vi "User Calibration.vi"(0 "CalStatusTab":T4(tab), 1 "SetDac In Process":bool, 5 "Processed Variables":T3 {"Chamber Temperature" format="%.2f"; "Ambient Temperature" format="%.2f"; "Bath Temperature" format="%.2f"; "Det. Temperature" format="%.2f"; "Detector Chl 4" format="%.2g"; "Detector Chl 3" format="%.2g"; "Ref CO2" format="%.2g"; "Detector Chl 2" format="%.2g"; "Film Temperature" format="%.2f"; "Humidity" format="%.2f"; "Detector Chl 1" format="%.2g"}, 9 "DACSet":u16[](array[numeric]) format="%03x", 11 "time_now":timestamp format="%<%H:%M:%S>T", 12 "Coefficients_In":T2[](array[typedef]) {"Elapsed Time" format="%<%H:%M:%S>t"; "zero_utc" format="%x"; "cal_utc" format="%x"; "Pump Flow Rate" format="%0d"; "Number of Zeroes" format="%0d"; "V2C" format="%0d"; "C2V" format="%0d"; "duration" format="%<%H:%M:%S>t"; "DAC" format="%03x"; "mI" format="%.3g"; "V_(RA,15mA)" format="%0.4f"; "V_(RA,5mA)" format="%0.4f"; "Chamber Temp" format="%.1f"; "Humidity" format="%.1f"}) -> (2 "Cal Fail":bool, 3 "Calibration Complete":bool, 4 "CalStatus Out":u16, 6 "DAC Currents":sgl[](array[numeric]) caption="Currents" format="%.4g", 8 "CalGasTank":u8=5 max=7, 10 "Pump Settings":T1, 14 "Coefficients_Out":T2[](array[typedef]) {"Elapsed Time" format="%<%H:%M:%S>t"; "zero_utc" format="%x"; "cal_utc" format="%x"; "Pump Flow Rate" format="%0d"; "Number of Zeroes" format="%0d"; "V2C" format="%0d"; "C2V" format="%0d"; "duration" format="%<%H:%M:%S>t"; "DAC" format="%03x"; "mI" format="%.3g"; "V_(RA,15mA)" format="%0.4f"; "V_(RA,5mA)" format="%0.4f"; "Chamber Temp" format="%.1f"; "Humidity" format="%.1f"}, 15 "SetDac":bool)   [LabVIEW 2015]
uses:
  <vilib>/Analysis/NI_AALBase.lvlib
  <vilib>/Analysis/baseanly.llb/Mean (DBL).vi
  Controls/Calibration Coefficients.ctl
  Controls/Processed Variables.ctl
  Controls/Pump Settings.ctl
panel:
  out "Error":bool
  out "Index":u16
  out "null array":i16[][](array[numeric])
  out "stage 4 - offset adjust":i16[][](array[numeric])=[[0, 3, 500, 1, 1], [1, 3, 500, 1, 1], [2, 3, 500, 1, 1], [3, 3, 500, 1, 1], [4, 3, 500, 1, 1], [5, 3, 500, 1, 1], [6, 3, 500, 1, 1], [7, 3, 500, 0, 0], [8, 3, 500, 0, 0], [9, 3, 500, 0, 0], [10, 3, 500, 0, 0], [11, 3, 500, 0, 0], [12, 3, 500, 0, 0], [13, 3, 500, 0, 0], [14, 3, 500, 0, 0], [15, 3, 500, 0, 0], [16, 3, 500, 0, 0], [17, 3, 500, 0, 0], [18, 3, 500, 0, 0], [19, 3, 500, 0, 0], [20, 3, 500, 0, 0], [21, 3, 500, 0, 0], [22, 3, 500, 0, 0], [23, 3, 500, 0, 0], [24, 3, 500, 0, 0], [25, 3, 500, 0, 0], [26, 3, 500, 0, 0], [27, 3, 500, 0, 0], [28, 3, 500, 0, 0], [29, 3, 500, 0, 0], [30, 3, 500, 0, 0], [31, 3, 500, 0, 0], [32, 3, 500, 0, 0], [33, 3, 500, 0, 0], [34, 3, 500, 0, 0], [35, 3, 500, 0, 0], [36, 3, 500, 0, 0], [37, 3, 500, 0, 0], [38, 3, 500, 0, 0], [39, 3, 500, 0, 0], [40, 3, 500, 0, 0], [41, 3, 500, 0, 0], [42, 3, 500, 0, 0], [43, 3, 500, 0, 0], [44, 3, 500, 0, 0], [45, 3, 500, 0, 0], [46, 3, 500, 0, 0], [47, 3, 500, 0, 0], [48, 3, 500, 0, 0], [49, 3, 500, 0, 0], [50, 3, 500, 0, 0], [51, 3, 500, 0, 0], [52, 3, 500, 0, 0], [53, 3, 500, 0, 0], [54, 3, 500, 0, 0], [55, 3, 500, 0, 0], [56, 3, 500, 0, 0], [57, 3, 500, 0, 0], [58, 3, 500, 0, 0], [59, 3, 500, 0, 0], [60, 3, 500, 0, 0], [61, 3, 500, 0, 0], [62, 3, 500, 0, 0], [63, 3, 500, 0, 0], [64, 3, 500, 0, 0], [65, 3, 500, 0, 0], [66, 3, 500, 0, 0], [67, 3, 500, 0, 0], [68, 3, 500, 0, 0], [69, 3, 500, 0, 0], [70, 3, 500, 0, 0], [71, 3, 500, 0, 0], [72, 3, 500, 0, 0], [73, 3, 500, 0, 0], [74, 3, 500, 0, 0], [75, 3, 500, 0, 0], [76, 3, 500, 0, 0], [77, 3, 500, 0, 0], [78, 3, 500, 0, 0], [79, 3, 500, 0, 0], [80, 3, 500, 0, 0], [81, 3, 500, 0, 0], [82, 3, 500, 0, 0], [83, 3, 500, 0, 0], [84, 3, 500, 0, 0], [85, 3, 500, 0, 0], [86, 3, 500, 0, 0], [87, 3, 500, 0, 0], [88, 3, 500, 0, 0], [89, 3, 500, 0, 0], [90, 3, 500, 0, 0], [91, 3, 500, 0, 0], [92, 3, 50, 1, 1]]
  out "stage 3 - span":i16[][](array[numeric])=[[0, 3, 500, 0, 1], [1, 3, 500, 0, 1], [2, 3, 500, 0, 1], [3, 3, 500, 0, 1], [4, 3, 500, 0, 1], [5, 3, 500, 0, 1], [6, 3, 50, 0, 1]]
  out "stage 2 - zeroing":i16[][](array[numeric])=[[0, 2, 500, 1, 0], [1, 2, 500, 1, 0], [2, 2, 500, 1, 0], [3, 2, 500, 1, 0], [4, 2, 500, 1, 0], [5, 2, 500, 1, 0], [6, 2, 50, 1, 0]]
  out "stage1 - humidity check":i16[][](array[numeric])=[[0, 1, 500, 1, 0], [1, 1, 50, 1, 0], [2, 1, 50, 1, 0], [3, 1, 50, 1, 0], [4, 1, 50, 1, 0], [5, 1, 50, 1, 0], [6, 1, 100, 0, 1], [7, 1, 150, 0, 1], [8, 1, 200, 0, 1], [9, 1, 250, 1, 0], [10, 1, 300, 1, 1], [0, 1, 350, 0, 0]]
  out "Tcal_Film":dbl format="%.2f"
  out "I_delta":dbl[](array[numeric]) format="%0.4f"
  out "Actual":u16
  in  "Lo Flow":u16=50
  out "Tcal_Det":dbl[](array[numeric]) format="%.2f"
  out "Raw_Humidity":dbl format="%.2f"
  out "Raw Chamber":dbl format="%.2f"
  in  "Quit":bool
  in  "CalFile":path
  in  "Calfiles":string[](array[string])
  out "Reference":dbl format="%.3g"
  out "Tcal_Humidity":dbl format="%.2f"
  in  "Hi Flow Setting":u16=100
  out "Progress Out":u8(slide) scale=0.0..255.0
  in  "Progress":u16(slide) scale=0.0..666.0
  out "Cal Gas":dbl=nan format="%.3g"
  in  "Skip Cal":bool
  in  "OK  7":bool
  in  "Calgas":dbl caption="Calibration Gas Concentration" format="%.2g"
  out "start time":timestamp format="%<%H:%M:%S>T"
  in  "Gas Tank":u8=5
  out "Calibration Message":enum16{"Calibration Is Required - "}(ring)
  in  "Calibration Code":T5(ring)
  out "Stable":bool
  in  "Low Humidity Threshold (%)":u16=60
  in  "Hi Humidity Threshold (%)":u16=90
  in  "Humidity Status":T6(ring)
  out "Stablizing":dbl[][](graph)
  out "Status":bool[](array[boolean])
  out "V2C":u8[](array[numeric])
  out "D'":dbl[](array[numeric]) format="%0.4f"
  out "C'":dbl[](array[numeric]) format="%0.4f"
  out "B'":dbl[](array[numeric]) format="%0.4f"
  out "A'":dbl[](array[numeric]) format="%0.4f"
  out "D":dbl[](array[numeric]) format="%0.4f"
  out "C":dbl[](array[numeric]) format="%0.4f"
  out "B":dbl[](array[numeric]) format="%0.4f"
  out "A":dbl[](array[numeric]) format="%0.4f"
  out "C2V":u8[](array[numeric])
  out "CHANNEL":string[](array[string])
  out "C0FC2V":dbl[](array[numeric]) format="%0.4f"
  out "C6FC2V":dbl[](array[numeric]) format="%0.4f"
  out "TYPE":string
  out "DATE":string
  out "CalFile Selected":path
  out "V_0d(target)":dbl[](array[numeric]) format="%0.4f"
  out "V_6d(target)":dbl[](array[numeric]) format="%0.4f"
  out "V_span(target)":dbl[](array[numeric]) format="%0.4f"
  out "BlueLED 2":bool[](array[boolean]) caption="BlueLED"
  out "DAC scale":dbl[](array[numeric]) format="%.3g"
  out "Zero":dbl[][](graph)
  out "Zero Status":T7(ring)
  out "V_RA(5mA)":dbl[](array[numeric]) format="%0.4f"
  out "V_RA(15mA)":dbl[](array[numeric]) format="%0.4f"
  out "mI":dbl[](array[numeric]) format="%.3g"
  out "delta 2":dbl=nan caption="delta" format="%.3g"
  out "CHANNEL 2":string[](array[string]) caption="CHANNEL"
  out "BlueLED":bool[](array[boolean])
  in  "OK 9":bool
  out "Span Point Calibration":dbl[][](graph)
  out "I_span":dbl[](array[numeric]) format="%0.4f"
  out "Step":i16[](array[numeric])
  out "DAC":u16[](array[numeric]) format="%03x"
  out "V_Span Delta":dbl[](array[numeric]) format="%0.4f"
  out "Span Good":bool[](array[boolean])
  out "I'mBlue":bool[](array[boolean]) caption="BlueLED"
  out "delta":dbl=nan format="%.3g"
  out "Zero Offset":dbl[][](graph)
  in  "OK 10":bool
  out "Calibration Complete -":timestamp format="%<%H:%M:%S\n%m/%d/%y>T"
  out "duration":i16 caption="mins" format="%<%H:%M:%S>t"
  out "V_0d(ImA)":dbl[](array[numeric]) format="%0.4f"
  out "V_6d(ImA)":dbl[](array[numeric]) format="%0.4f"
  out "V_0(adjust)":dbl[](array[numeric]) format="%0.4f"
  out "V_span(adjust)":dbl[](array[numeric]) format="%0.4f"
  out "Gain(adjust)":dbl[](array[numeric]) format="%0.4f"
  out "V_span(ImA)":dbl[](array[numeric]) format="%0.4f"
  out "Tcal_PCB":dbl=nan format="%.2f"
  out "Tcal_Chamber":dbl format="%.2f"
  out "elapsed time":i16 format="%<%H:%M:%S>t"
  out "Count":u8
  # "Channel 1"
  # "Channel 2"
  # "Channel 3"
  # "Channel 4"
  # "Initializing"
  # "1. Please Place Freespira On Base-Station\n \n2. Attach Cannula and Breathe Normally \n \n3. Enter Calibration Gas Concentration \n \n4. Press OK To Begin Calibration Process"
  # "Please Enter Calibration Code"
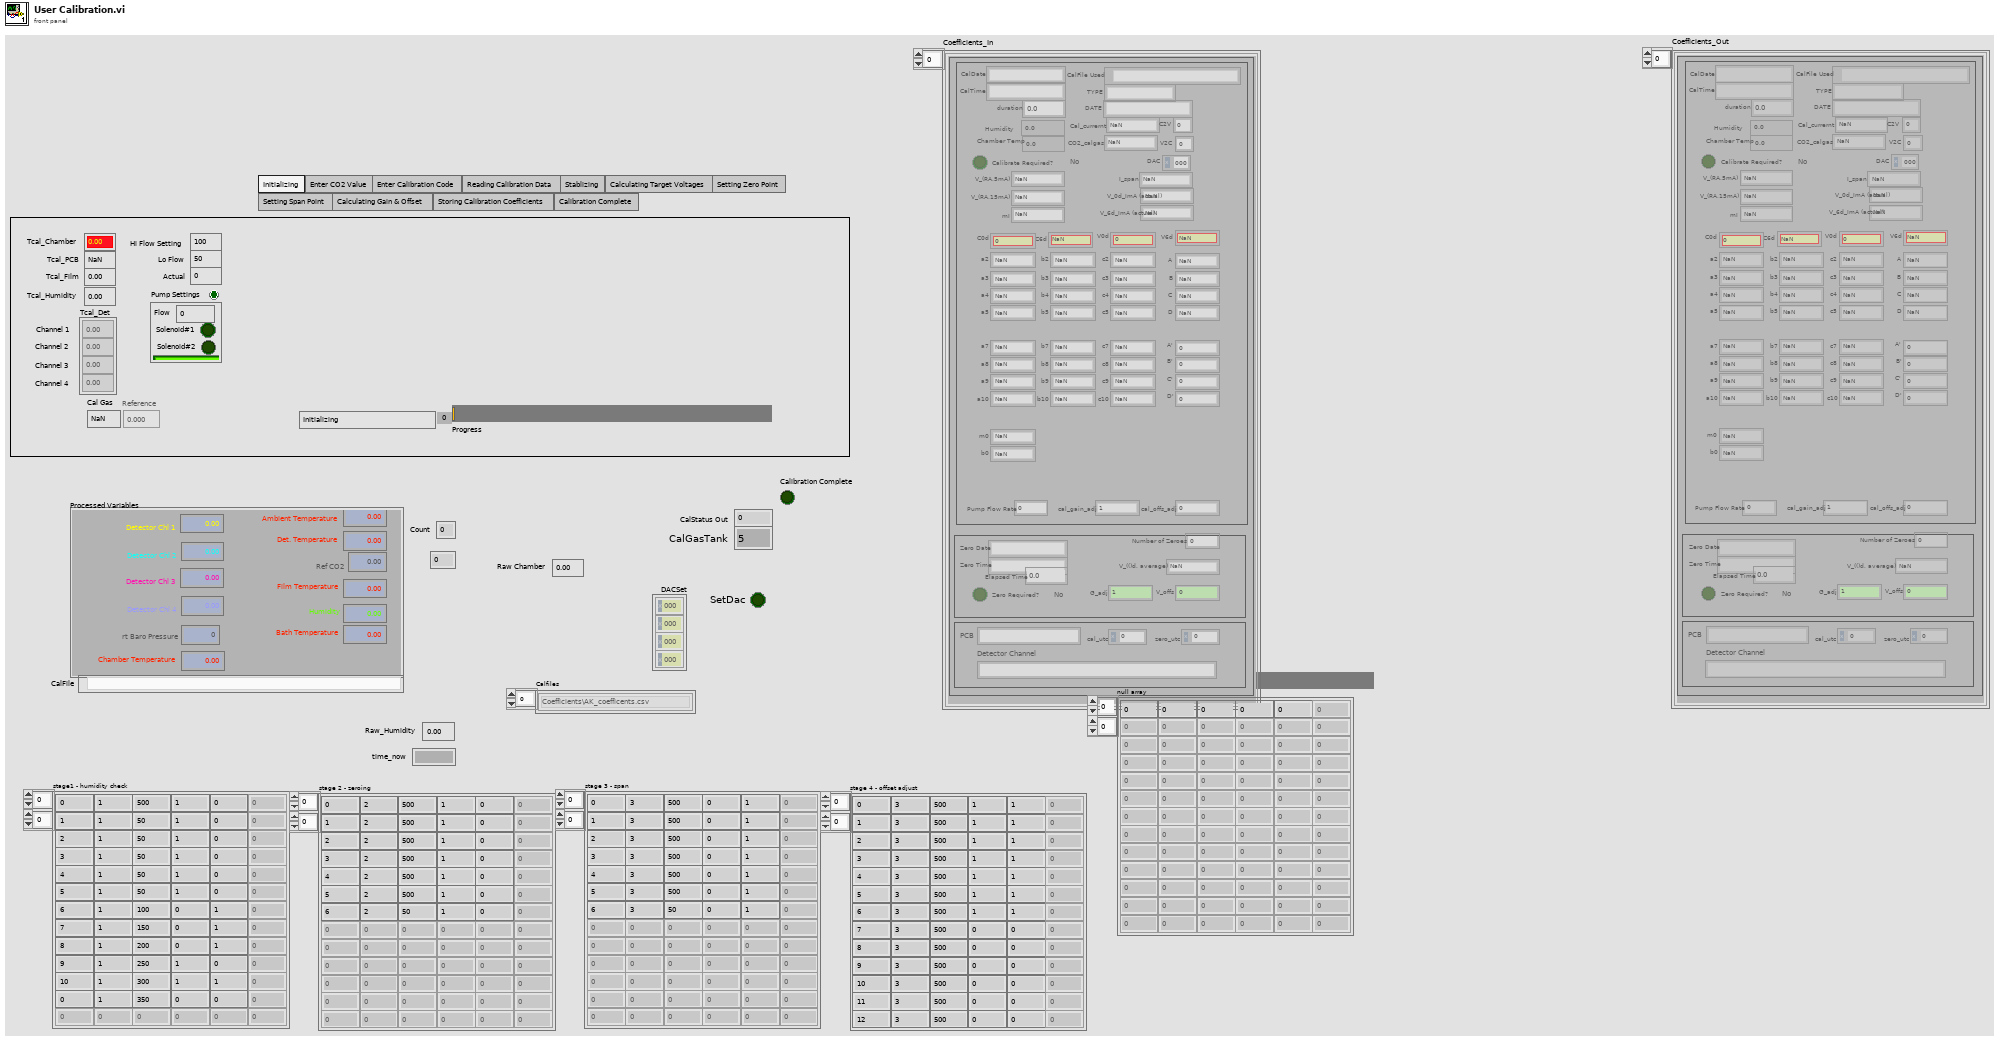
[diagram p1: front panel]
types:
  T1 = typedef "Pump Settings.ctl" = cluster{"Flow":u16, "Solenoid#1":bool, "Solenoid#2":bool, "ignore":bool}
  T2 = typedef "Calibration Coefficients.ctl" = cluster{"CalFile Used":path, "TYPE":string, "DATE":string, "Humidity":sgl, "Chamber Temp":dbl, "CO2_calgas":dbl, "V_(RA,5mA)":dbl, "V_(RA,15mA)":dbl, "mI":dbl, "V_0d_ImA (actual)":dbl, "V_6d_ImA (actual)":dbl, "I_span":dbl, "DAC":u16, "A":dbl, "B":dbl, "C":dbl, "D":dbl, "V6d":dbl, "A'":dbl, "B'":dbl, "C'":dbl, "D'":dbl, "V0d":dbl, "CalDate":string, "CalTime":string, "duration":dbl, "Detector Channel":string, "a2":dbl, "a3":dbl, "a4":dbl, "a5":dbl, "b2":dbl, "c2":dbl, "b3":dbl, "c3":dbl, "b4":dbl, "c4":dbl, "b5":dbl, "c5":dbl, "a7":dbl, "a8":dbl, "a9":dbl, "a10":dbl, "b7":dbl, "b8":dbl, "b9":dbl, "b10":dbl, "c7":dbl, "c8":dbl, "c9":dbl, "c10":dbl, "cal_offs_adj":dbl, "cal_gain_adj":dbl, "C6d":dbl, "C0d":dbl, "Cal_currernt":dbl, "C2V":u16, "V2C":u16, "Zero Date":string, "Zero Time":string, "Number of Zeroes":u16, "V_(()d, average)":dbl, "V_offs ":dbl, "G_adj":dbl, "Pump Flow Rate":u16, "Zero Required? ":bool, "Calibrate Required?":bool, "cal_utc":dbl, "zero_utc":dbl, "Elapsed Time":dbl, "PCB":string, "m0":dbl, "b0":dbl}
  T3 = typedef "Processed Variables.ctl" = cluster{"Detector Chl 1":sgl, "Humidity":dbl, "Film Temperature":dbl, "Detector Chl 2":sgl, "Ref CO2":sgl, "Detector Chl 3":sgl, "Detector Chl 4":sgl, "Det. Temperature":dbl, "Bath Temperature":dbl, "Ambient Temperature":dbl, "rt Baro Pressure":u16, "Chamber Temperature":dbl}
  T4 = enum32{"Initializing", "Enter CO2 Value", "Enter Calibration Code", "Reading Calibration Data", "Stablizing", "Calculating Target Voltages", "Setting Zero Point", "Setting Span Point", "Calculating Gain & Offset", "Storing Calibration Coefficients", "Calibration Complete"}
  T5 = enum8{"", "<User Defined>", "11111 - default", "22222 - MM_1_NS", "33333 - MM_2_S"}
  T6 = enum16{"Waiting For Film to Stabilize", "Film Stable", "Exiting", "Initializing"}
  T7 = enum16{"Setting Zero at 5 mA", "Setting Zero at 15 mA", "Calculating slopes"}
  T8 = enum32{"Invalid", "Standard", "Closed", "Hidden", "Minimized", "Maximized"}
  T9 = enum16{"Waiting For Film to Stabilize", "Film Stable - Press OK to Continue", "Exiting"}
  T10 = enum16{"Waiting For Film to Stabilize", "Film Stable - Press OK to Continue", "Exiting", "Initializing"}
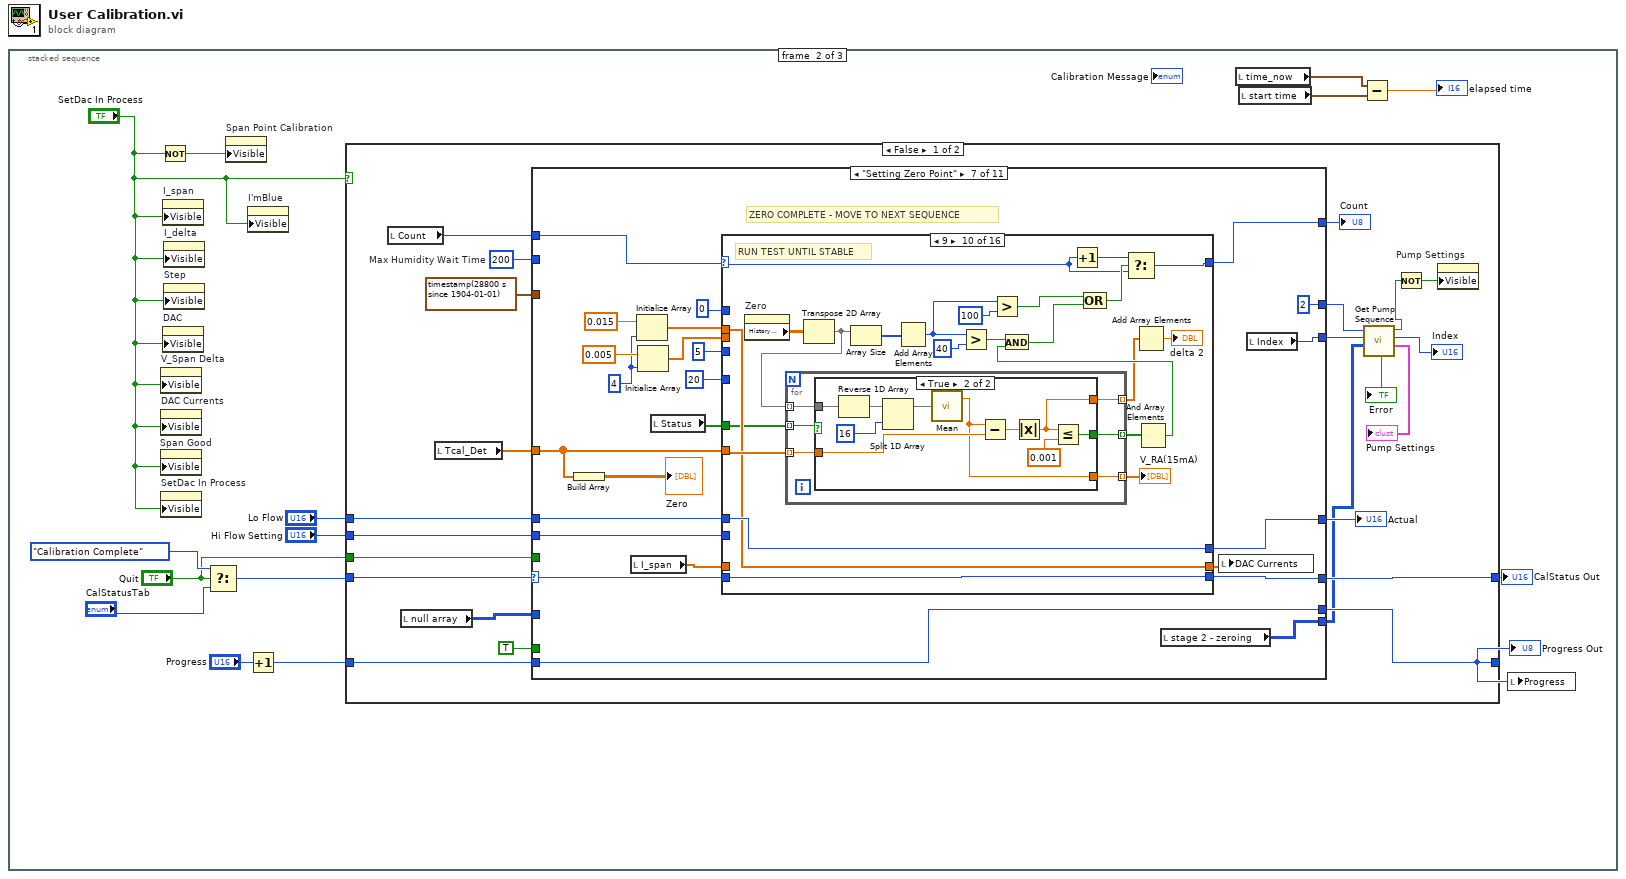
[diagram p0: block diagram]
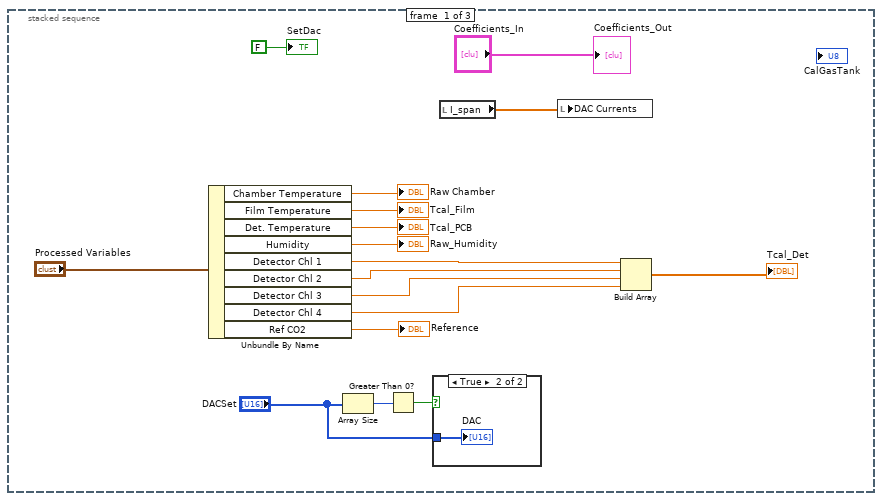
[diagram p2: hidden frame]
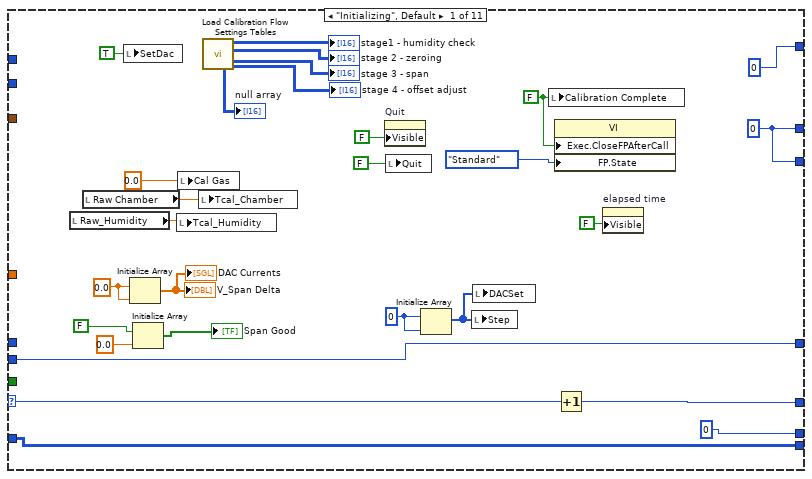
[diagram p4: hidden frame]
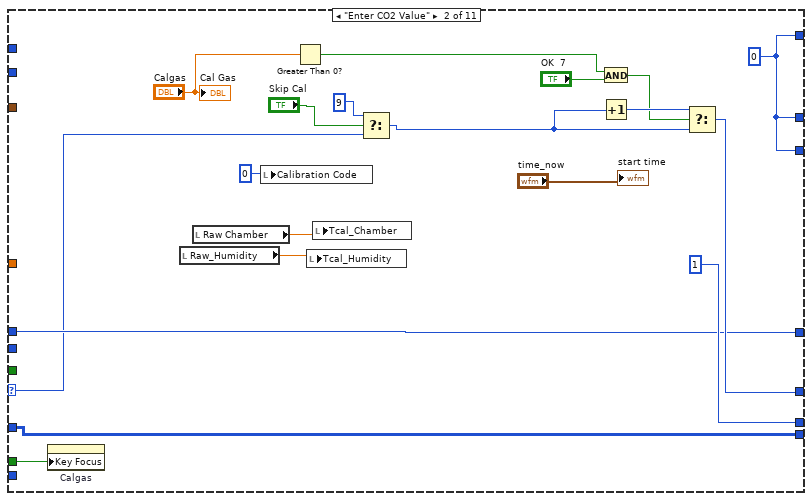
[diagram p5: hidden frame]
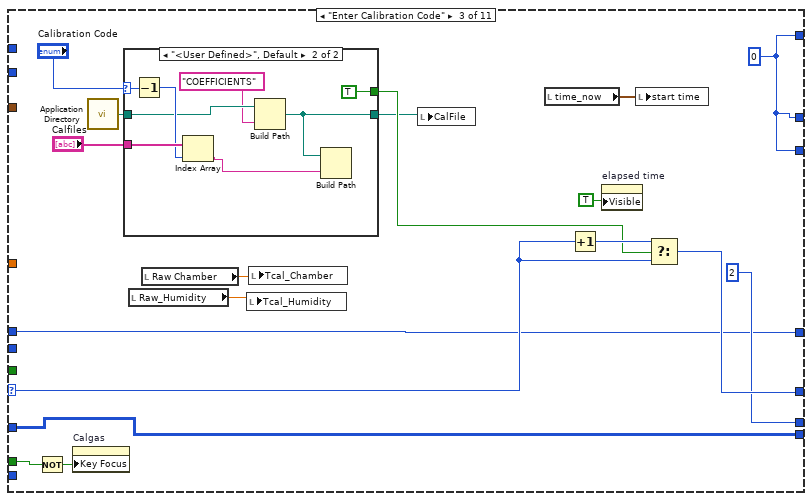
[diagram p6: hidden frame]
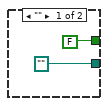
[diagram p7: hidden frame]
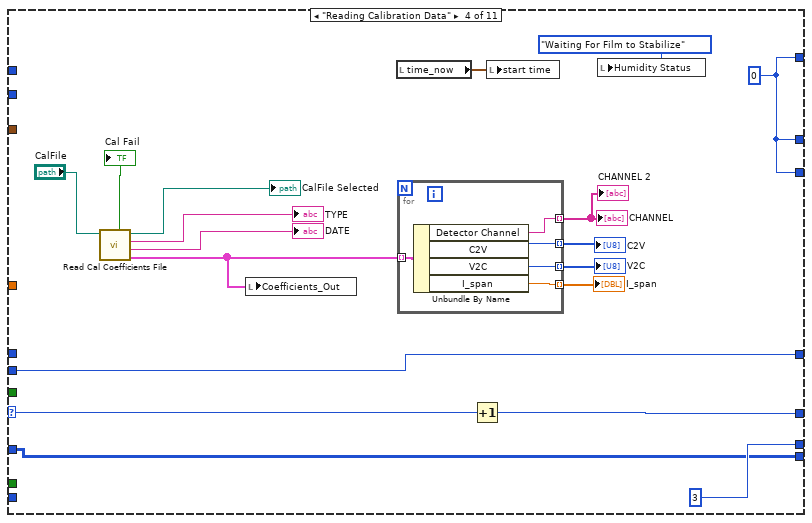
[diagram p8: hidden frame]
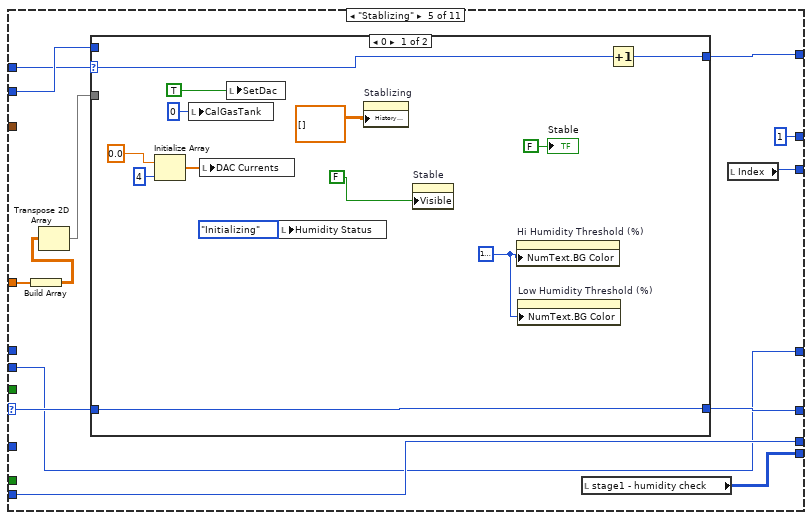
[diagram p9: hidden frame]
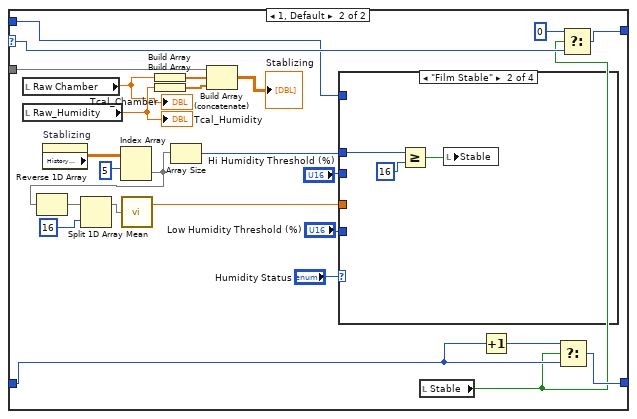
[diagram p10: hidden frame]
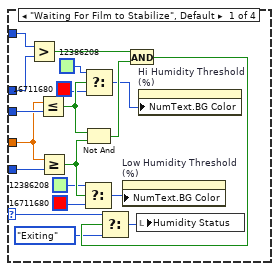
[diagram p11: hidden frame]
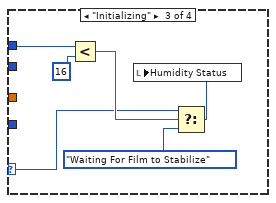
[diagram p12: hidden frame]
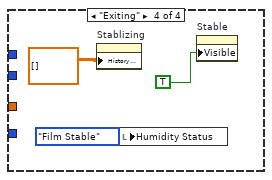
[diagram p13: hidden frame]
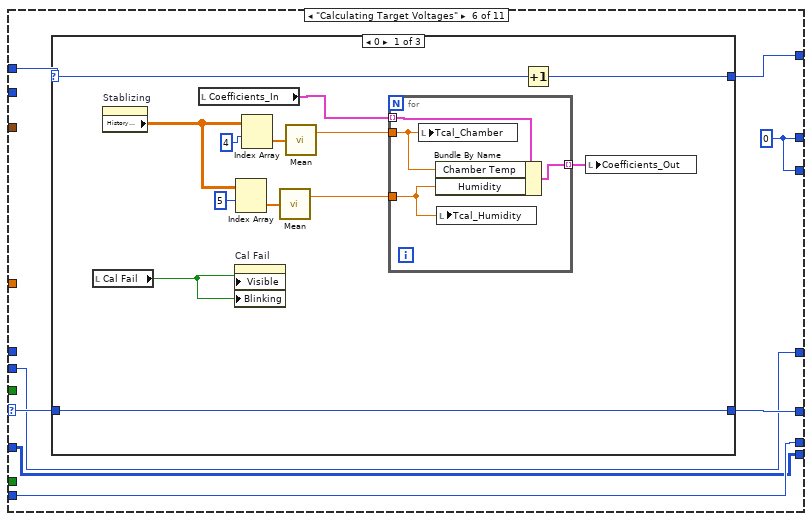
[diagram p14: hidden frame]
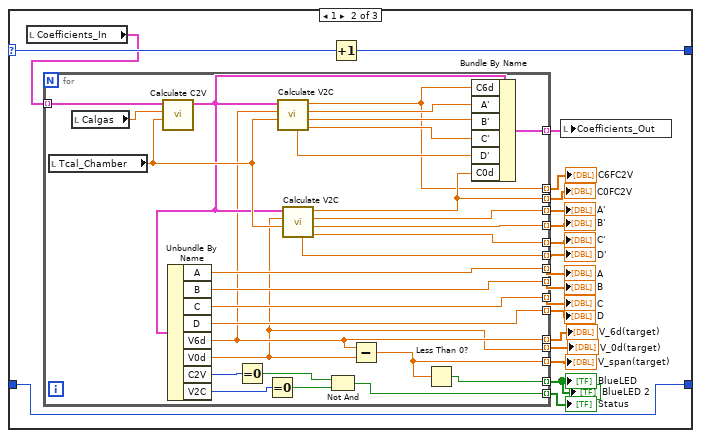
[diagram p15: hidden frame]
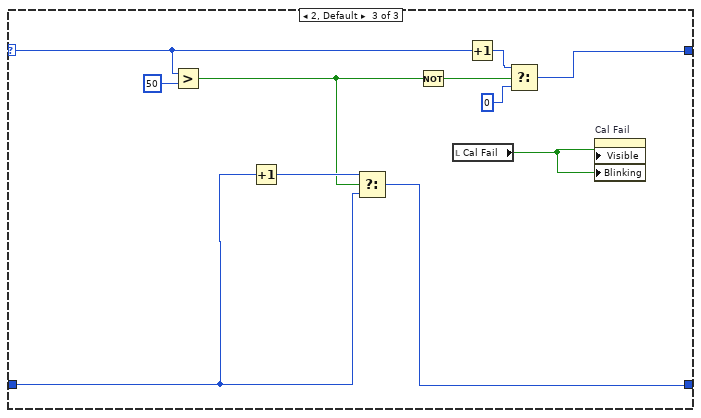
[diagram p16: hidden frame]
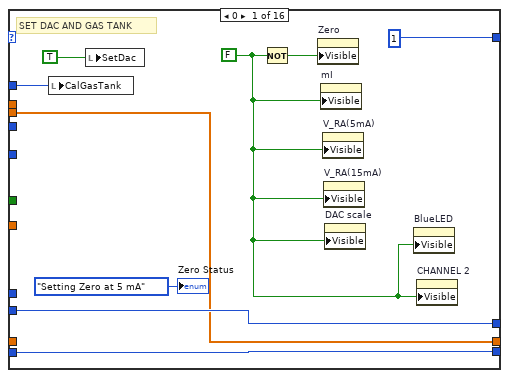
[diagram p17: hidden frame]
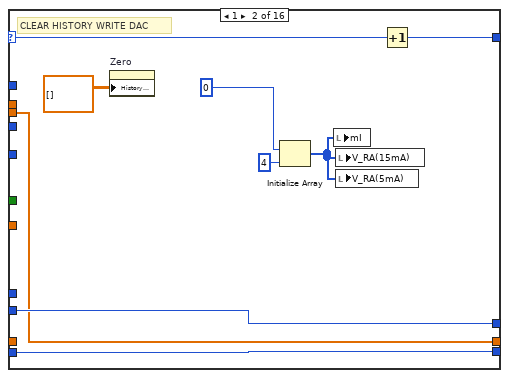
[diagram p18: hidden frame]
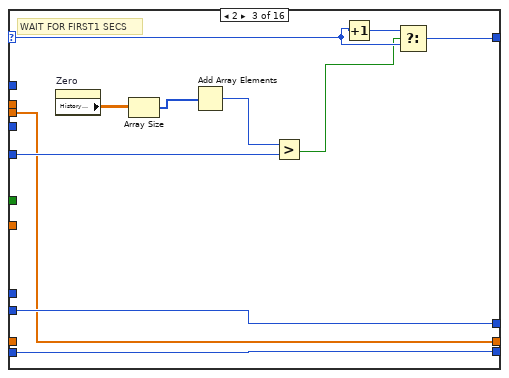
[diagram p19: hidden frame]
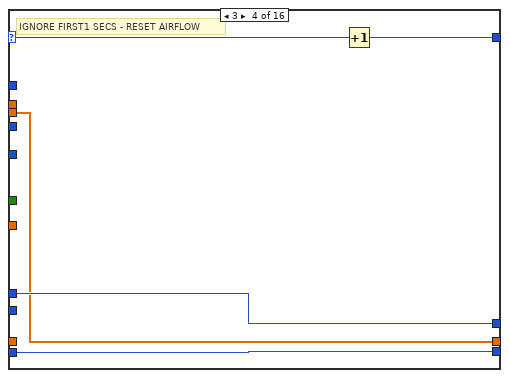
[diagram p20: hidden frame]
diagram:
  n1 = stacked-sequence {
    frame #0 {
      n2 = Unbundle By Name("Processed Variables") -> ("Chamber Temperature"=→"Raw Chamber":dbl, "Film Temperature"=→"Tcal_Film":dbl, "Det. Temperature"=→"Tcal_PCB":dbl, "Humidity"=→"Raw_Humidity":dbl, "Detector Chl 1"=w10:sgl, "Detector Chl 2"=w9:sgl, "Detector Chl 3"=w8:sgl, "Detector Chl 4"=w12:sgl, "Ref CO2"=→"Reference":sgl)
      n3 = Array Size(array="DACSet") -> (size(s)=w6:i32)
      n4 = Greater Than 0?(x=w6) -> (x > 0?=w5:bool)
      n5 = case shown="True" w5 {
        tunnel: "DACSet" -> [_ w18]
        frame False {
        }
        frame True {
          "DAC" <- w18
        }
      }
      n6 = local read "I_span"() -> (w4:dbl[])
      n7 = local write "DAC Currents"(w4) -> ()
      n8 = Build Array(w10, w9, w8, w12) -> (→"Tcal_Det":sgl[])
      "SetDac" <- FALSE
      "Coefficients_Out" <- "Coefficients_In"
    }
    frame #1 {
      n9 = Not(x="SetDac In Process") -> (.not. x?=w20:bool)
      n10 = property on="V_Span Delta" class="Arr (strict)"("Visible"="SetDac In Process") -> ()  [unwired: 2 in, 2 out]
      n11 = property on="DAC Currents" class="Arr (strict)"("Visible"="SetDac In Process") -> ()  [unwired: 2 in, 2 out]
      n12 = property on="Span Good" class="Arr (strict)"("Visible"="SetDac In Process") -> ()  [unwired: 2 in, 2 out]
      n13 = property on="SetDac In Process" class="Bool (strict)"("Visible"="SetDac In Process") -> ()  [unwired: 2 in, 2 out]
      n14 = property on="I_span" class="Arr (strict)"("Visible"="SetDac In Process") -> ()  [unwired: 2 in, 2 out]
      n15 = property on="DAC" class="Arr (strict)"("Visible"="SetDac In Process") -> ()  [unwired: 2 in, 2 out]
      n16 = property on="I_delta" class="Arr (strict)"("Visible"="SetDac In Process") -> ()  [unwired: 2 in, 2 out]
      n17 = property on="Step" class="Arr (strict)"("Visible"="SetDac In Process") -> ()  [unwired: 2 in, 2 out]
      n18 = Select(t=T4."Calibration Complete" ("CalStatusTab"), s="Quit", f="CalStatusTab") -> (s? t:f=w24:T4)
      n19 = property on="Span Point Calibration" class="WFChart (strict)"("Visible"=w20) -> ()  [unwired: 2 in, 2 out]
      n20 = property on="I'mBlue" class="Arr (strict)"("Visible"="SetDac In Process") -> ()  [unwired: 2 in, 2 out]
      n21 = Increment(x="Progress") -> (x+1=w23:u16)
      n22 = case shown="False" "SetDac In Process" {
        tunnel: [w56 w1090] -> w33
        tunnel: [w55 w1089] -> w31
        tunnel: "Quit" -> [w51 _]
        tunnel: w24 -> [w50 w1089]
        tunnel: w23 -> [w49 w1090]
        tunnel: "Lo Flow" -> [w45 _]
        tunnel: "Hi Flow Setting" -> [w44 _]
        frame False {
          w54 = 200  # Max Humidity Wait Time
          n23 = local read "Count"() -> (w53:u8)
          n24 = local read "null array"() -> (w42:i16[][])
          n25 = local read "Tcal_Det"() -> (w47:dbl[])
          n26 = case shown="\"Setting Zero Point\"" w50 {
            selector: w50 -> [w84 w93 w118 w149 w165 w244 w344 w592 w899 w999 w1084]
            tunnel: [w80 w103 w121 w147 w164 w243 w343 w591 w898 w998 w1084] -> w55
            tunnel: w49 -> [_ _ _ _ w163 w239 w342 w590 w900 w997 w1083]
            tunnel: [0 1 2 3 w163 w239 w342 w590 w900 w996 w1082] -> w56
            tunnel: w51 -> [_ _ _ _ _ _ _ _ _ _ _]
            tunnel: w45 -> [_ w96 w113 _ _ _ w337 w586 w893 w995 w1080]
            tunnel: w44 -> [w77 _ _ w144 w159 w240 w336 w585 w894 _ _]
            tunnel: w54 -> [_ _ _ _ w166 _ _ _ _ _ _]
            tunnel: w53 -> [_ _ _ _ w158 w242 w324 w573 w887 w994 w1081]
            tunnel: [u8 0 w85 w104 w132 w167 w241 w338 w587 w897 w993 w1081] -> w48
            tunnel: [w77 w96 w113 w144 w159 w240 w335 w584 w896 w992 w1080] -> w46
            tunnel: timestamp(28800 s since 1904-01-01) -> [_ _ _ _ _ _ _ _ _ w991 _]
            tunnel: w47 -> [_ _ _ _ w162 _ w334 w582 w891 _ _]
            tunnel: TRUE ("Key Focus") -> [_ w87 w109 _ _ _ _ _ _ _ _]
            tunnel: [w58 w86 w105 w133 w157 w238 w323 w572 w888 w990 w1078] -> w38
            tunnel: w42 -> [w58 w86 w105 w133 _ w238 _ _ _ w990 w1078]
            tunnel: [w57 w85 w104 w132 1 w237 2 ("Count") 3 ("Count") 4 ("Count") w989 w1077] -> w41
            tunnel: [w57 w85 w104 w132 w156 w237 w321 w571 w886 w989 w1077] -> w40
            frame "Initializing", Default {
              w57 = 0
              w70 = 0.0
              w72 = 0
              w82 = FALSE ("Calibration Complete")
              n27 = local read "Raw_Humidity"() -> (w75:dbl)
              n28 = local read "Raw Chamber"() -> (w74:dbl)
              n29 = local write "SetDac"(TRUE ("SetDac")) -> ()
              n30 = Initialize Array(w70, w70) -> (→"V_Span Delta" →"DAC Currents":dbl[])
              n31 = Initialize Array(FALSE, 0.0) -> (→"Span Good":bool[])
              n32 = local write "Tcal_Humidity"(w75) -> ()
              n33 = local write "Cal Gas"(0.0) -> ()
              n34 = local write "Tcal_Chamber"(w74) -> ()
              n35 = call "Load Calibration Flow Settings Tables.vi"() -> ("stage 4 - span"=→"stage 4 - offset adjust":i16[][], "stage 3 - high"=→"stage 3 - span":i16[][], "stage 2 - zeroing"=→"stage 2 - zeroing":i16[][], "stage1 - humidity check"=→"stage1 - humidity check":i16[][], "stage 5 - offset adjust"=→"null array":i16[][])  [unwired: 6 in, 1 out]
              n36 = property on="Quit" class="Bool (strict)"("Visible"=FALSE ("Blinking")) -> ()  [unwired: 2 in, 2 out]
              n37 = local write "Quit"(FALSE ("Cal Fail")) -> ()
              n38 = Initialize Array(w72, w72) -> (w65:i32[])
              n39 = local write "Step"(w65) -> ()
              n40 = local write "DACSet"(w65) -> ()
              n41 = local write "Calibration Complete"(w82) -> ()
              n42 = property class="VI"("Exec.CloseFPAfterCall"=w82, "FP.State"=T8."Standard" ("Front Panel Window:State")) -> ()  [unwired: 2 in, 2 out]
              n43 = Increment(x=w84) -> (x+1=w80:T4)
              n44 = property on="elapsed time" class="DigNum (strict)"("Visible"=FALSE) -> ()  [unwired: 2 in, 2 out]
            }
            frame "Enter CO2 Value" {
              w85 = u8 0
              n45 = property on="Calgas" class="DigNum (strict)"("Key Focus"=w87) -> ()  [unwired: 2 in, 2 out]
              n46 = local read "Raw_Humidity"() -> (w90:dbl)
              n47 = local read "Raw Chamber"() -> (w89:dbl)
              n48 = local write "Calibration Code"(0) -> ()
              n49 = Greater Than 0?(x="Calgas") -> (x > 0?=w88:bool)
              n50 = local write "Tcal_Humidity"(w90) -> ()
              n51 = local write "Tcal_Chamber"(w89) -> ()
              n52 = Select(t=u16 9 ("CalStatus Out"), s="Skip Cal", f=w93) -> (s? t:f=w94:u32)
              n53 = And(x=w88, y="OK  7") -> (x .and. y?=w97:bool)
              n54 = Increment(x=w94) -> (x+1=w102:u32)
              n55 = Select(t=w102, s=w97, f=w94) -> (s? t:f=w103:u32)
              "start time" <- "time_now"
              "Cal Gas" <- "Calgas"
            }
            frame "Enter Calibration Code" {
              w104 = u8 0
              n56 = Not(x=w109) -> (.not. x?=w108:bool)
              n57 = property on="Calgas" class="DigNum (strict)"("Key Focus"=w108) -> ()  [unwired: 2 in, 2 out]
              n58 = call <vilib>:"Application Directory.vi"() -> ("Application Directory"=w107:path)
              n59 = case shown="\"<User Defined>\", Default" "Calibration Code" {
                selector: "Calibration Code" -> [_ w129]
                tunnel: [FALSE TRUE] -> w117
                tunnel: "Calfiles" -> [_ w130]
                tunnel: w107 -> [_ w126]
                tunnel: [path "" w124] -> w106
                frame "" {
                }
                frame "<User Defined>", Default {
                  n60 = Decrement(x=w129) -> (x-1=w128:T5)
                  n61 = Index Array(array=w130, index=w128) -> (element=w131:string)
                  n62 = Build Path(base path=w126, name or relative path="COEFFICIENTS") -> (appended path=w124:path)
                  n63 = Build Path(base path=w124, name or relative path=w131) -> ()  [unwired: 1 out]
                }
              }
              n64 = local read "Raw_Humidity"() -> (w112:dbl)
              n65 = local read "Raw Chamber"() -> (w111:dbl)
              n66 = local write "Tcal_Humidity"(w112) -> ()
              n67 = local write "Tcal_Chamber"(w111) -> ()
              n68 = local write "CalFile"(w106) -> ()
              n69 = local read "time_now"() -> (w110:timestamp)
              n70 = Increment(x=w118) -> (x+1=w120:T4)
              n71 = property on="elapsed time" class="DigNum (strict)"("Visible"=TRUE) -> ()  [unwired: 2 in, 2 out]
              n72 = local write "start time"(w110) -> ()
              n73 = Select(t=w120, s=w117, f=w118) -> (s? t:f=w121:T4)
            }
            frame "Reading Calibration Data" {
              w132 = u8 0
              n74 = call "Read Cal Coefficients File.vi"(11:"CalFile") -> ("Original Coefficients"=w140:T2[], "DATE"=→"DATE":string, "TYPE"=→"TYPE":string, "CalFile Selected"=→"CalFile Selected":path, "Error"=→"Cal Fail":bool)  [unwired: 5 in, 1 out]
              n75 = local write "Coefficients_Out"(w140) -> ()
              n76 = local read "time_now"() -> (w145:timestamp)
              n77 = for {
                tunnel: w140 -> [w154] mode=indexing
                tunnel: [w153] -> w137 mode=indexing
                tunnel: [w152] -> w136 mode=indexing
                tunnel: [w151] -> w135 mode=indexing
                tunnel: [w150] -> w134 mode=indexing
                n78 = Unbundle By Name(w154) -> ("Detector Channel"=w150:string, "C2V"=w151:u16, "V2C"=w152:u16, "I_span"=w153:dbl)
              }
              "I_span" <- w137
              "V2C" <- w136
              "C2V" <- w135
              "CHANNEL" <- w134
              "CHANNEL 2" <- w134
              n79 = Increment(x=w149) -> (x+1=w147:T4)
              n80 = local write "start time"(w145) -> ()
              n81 = local write "Humidity Status"(enum16{"Waiting For Film to Stabilize"}."Waiting For Film to Stabilize" ("Enum")) -> ()
            }
            frame "Stablizing" {
              n82 = Build Array(w162) -> (w161:dbl[][])
              n83 = Transpose 2D Array(2D array=w161) -> (transposed array=w160:dbl[][])
              n84 = case shown="0" w158 {
                selector: w158 -> [w180 w200]
                tunnel: [w179 w201] -> w167
                tunnel: w166 -> [_ w195]
                tunnel: w165 -> [w178 w199]
                tunnel: [w178 w198] -> w164
                tunnel: w160 -> [_ w182]
                frame 0 {
                  w172 = u32 16777216
                  n85 = Initialize Array(0.0, 4 ("dimension size")) -> (w170:dbl[])
                  n86 = local write "CalGasTank"(u8 0 ("CalGasTank")) -> ()
                  n87 = local write "DAC Currents"(w170) -> ()
                  n88 = local write "SetDac"(TRUE ("InCal")) -> ()
                  n89 = local write "Humidity Status"(T6."Initializing" ("Humidity Status")) -> ()
                  n90 = property on="Stablizing" class="WFChart (strict)"("History Data"=dbl[][] []) -> ()  [unwired: 2 in, 2 out]
                  n91 = property on="Stable" class="Bool (strict)"("Visible"=FALSE) -> ()  [unwired: 2 in, 2 out]
                  n92 = property on="Hi Humidity Threshold (%)" class="DigNum (strict)"("NumText.BG Color"=w172) -> ()  [unwired: 2 in, 2 out]
                  n93 = property on="Low Humidity Threshold (%)" class="DigNum (strict)"("NumText.BG Color"=w172) -> ()  [unwired: 2 in, 2 out]
                  n94 = Increment(x=w180) -> (x+1=w179:u8)
                  "Stable" <- FALSE ("Done")
                }
                frame 1, Default {
                  n95 = local read "Raw Chamber"() -> (w183:dbl)
                  "Tcal_Chamber" <- w183
                  n96 = local read "Raw_Humidity"() -> (w184:dbl)
                  "Tcal_Humidity" <- w184
                  n97 = property on="Stablizing" class="WFChart (strict)"() -> ("History Data"=w203:dbl[][])  [unwired: 2 in, 2 out]
                  n98 = Index Array(array=w203, index (row)=5) -> (element=w190:dbl[])  [unwired: 1 in]
                  n99 = Reverse 1D Array(array=w190) -> (reversed array=w191:dbl[])
                  n100 = Split 1D Array(array=w191, index=16) -> (first subarray=w192:dbl[])  [unwired: 1 out]
                  n101 = call-poly <vilib>:"Mean.vi"("X"=w192) -> ("mean"=w189:dbl)  [unwired: 1 out]
                  n102 = Build Array(w183) -> (w185:dbl[])
                  n103 = Build Array(w184) -> (w187:dbl[])
                  n104 = Array Size(array=w190) -> (size(s)=w197:i32)
                  n105 = Build Array (concatenate)(w182, w185, w187) -> (→"Stablizing":dbl[][])
                  n106 = case shown="\"Film Stable\"" "Humidity Status" {
                    selector: "Humidity Status" -> [w221 _ w228 _]
                    tunnel: w197 -> [w215 w227 w233 _]
                    tunnel: w195 -> [w216 _ _ _]
                    tunnel: "Hi Humidity Threshold (%)" -> [w223 _ _ _]
                    tunnel: "Low Humidity Threshold (%)" -> [w222 _ _ _]
                    tunnel: w189 -> [w217 _ _ _]
                    frame "Waiting For Film to Stabilize", Default {
                      n107 = Greater?(x=w216, y=w215) -> (0:w220:bool)
                      n108 = Less Or Equal?(x=w217, y=w223) -> (x <= y?=w210:bool)
                      n109 = Greater Or Equal?(x=w217, y=w222) -> (x >= y?=w212:bool)
                      n110 = Select(t=u32 12386208, s=w212, f=u32 16711680) -> (s? t:f=w213:u32)
                      n111 = Select(t=u32 12386208, s=w210, f=u32 16711680) -> (s? t:f=w211:u32)
                      n112 = Not And(1:w212, 2:w210) -> (0:w218:bool)
                      n113 = property on="Low Humidity Threshold (%)" class="DigNum (strict)"("NumText.BG Color"=w213) -> ()  [unwired: 2 in, 2 out]
                      n114 = And(x=w220, y=w218) -> (x .and. y?=w219:bool)
                      n115 = Select(t=w221, s=w219, f=T9."Exiting" ("Humidity Status")) -> (s? t:f=w224:u16)
                      n116 = local write "Humidity Status"(w224) -> ()
                      n117 = property on="Hi Humidity Threshold (%)" class="DigNum (strict)"("NumText.BG Color"=w211) -> ()  [unwired: 2 in, 2 out]
                    }
                    frame "Film Stable" {
                      n118 = Greater Or Equal?(x=w227, y=16) -> (x >= y?=w225:bool)
                      n119 = local write "Stable"(w225) -> ()
                    }
                    frame "Initializing" {
                      n120 = Less?(x=w233, y=16) -> (x < y?=w231:bool)
                      n121 = Select(t=w228, s=w231, f=T10."Waiting For Film to Stabilize" ("Humidity Status")) -> (s? t:f=w230:u16)
                      n122 = local write "Humidity Status"(w230) -> ()
                    }
                    frame "Exiting" {
                      n123 = property on="Stablizing" class="WFChart (strict)"("History Data"=dbl[][] []) -> ()  [unwired: 2 in, 2 out]
                      n124 = local write "Humidity Status"(T6."Film Stable" ("Humidity Status")) -> ()
                      n125 = property on="Stable" class="Bool (strict)"("Visible"=TRUE) -> ()  [unwired: 2 in, 2 out]
                    }
                  }
                  n126 = local read "Stable"() -> (w181:bool)
                  n127 = Increment(x=w199) -> (x+1=w202:T4)
                  n128 = Select(t=w202, s=w181, f=w199) -> (s? t:f=w198:T4)
                  n129 = Select(t=u8 0, s=w181, f=w200) -> (s? t:f=w201:u8)
                }
              }
              n130 = local read "stage1 - humidity check"() -> (w157:i16[][])
              n131 = local read "Index"() -> (w156:u16)
            }
            frame "Calculating Target Voltages" {
              w237 = u8 0 ("Count")
              n132 = case shown="0" w242 {
                selector: w242 -> [w249 w281 w320]
                tunnel: w244 -> [w250 w264 w318]
                tunnel: [w250 w264 w317] -> w243
                tunnel: [w248 w278 w312] -> w241
                frame 0 {
                  n133 = local read "Cal Fail"() -> (w245:bool)
                  n134 = property on="Stablizing" class="WFChart (strict)"() -> ("History Data"=w253:dbl[][])  [unwired: 2 in, 2 out]
                  n135 = local read "Coefficients_In"() -> (w247:T2[])
                  n136 = property on="Cal Fail" class="Bool (strict)"("Visible"=w245, "Blinking"=w245) -> ()  [unwired: 2 in, 2 out]
                  n137 = Index Array(array=w253, index (row)=5) -> (element=w255:dbl[])  [unwired: 1 in]
                  n138 = Index Array(array=w253, index (row)=4) -> (element=w256:dbl[])  [unwired: 1 in]
                  n139 = call-poly <vilib>:"Mean.vi"("X"=w255) -> ("mean"=w251:dbl)  [unwired: 1 out]
                  n140 = call-poly <vilib>:"Mean.vi"("X"=w256) -> ("mean"=w252:dbl)  [unwired: 1 out]
                  n141 = for {
                    tunnel: w252 -> [w261]
                    tunnel: [w260] -> w246 mode=indexing
                    tunnel: w251 -> [w259]
                    tunnel: w247 -> [w258] mode=indexing
                    n142 = local write "Tcal_Chamber"(w261) -> ()
                    n143 = Bundle By Name(cluster=w258, "Chamber Temp"=w261, "Humidity"=w259) -> (w260:T2)
                    n144 = local write "Tcal_Humidity"(w259) -> ()
                  }
                  n145 = Increment(x=w249) -> (x+1=w248:u8)
                  n146 = local write "Coefficients_Out"(w246) -> ()
                }
                frame 1 {
                  n147 = local read "Coefficients_In"() -> (w280:T2[])
                  n148 = for {
                    tunnel: w280 -> [w307] mode=indexing
                    tunnel: [w306] -> w279 mode=indexing
                    tunnel: [w283] -> w277 mode=indexing
                    tunnel: [w290] -> w266 mode=indexing
                    tunnel: [w305] -> w276 mode=indexing
                    tunnel: [w304] -> w275 mode=indexing
                    tunnel: [w303] -> w274 mode=indexing
                    tunnel: [w298] -> w273 mode=indexing
                    tunnel: [w302] -> w269 mode=indexing
                    tunnel: [w301] -> w270 mode=indexing
                    tunnel: [w300] -> w271 mode=indexing
                    tunnel: [w299] -> w272 mode=indexing
                    tunnel: [w297] -> w268 mode=indexing
                    tunnel: [w291] -> w267 mode=indexing
                    tunnel: [w289] -> w265 mode=indexing
                    tunnel: [w284] -> w263 mode=indexing
                    tunnel: [w282] -> w262 mode=indexing
                    n149 = local read "Tcal_Chamber"() -> (w309:dbl)
                    n150 = local read "Calgas"() -> (w308:dbl)
                    n151 = call "Calculate C2V.vi"("Tcal_Chamber"=w309, "CO2"=w308, "Calibration Coefficients"=w307) -> ("Calibration Coefficients Out"=w292:T2)  [unwired: 8 in]
                    n152 = Unbundle By Name(w292) -> ("A"=w298:dbl, "B"=w303:dbl, "C"=w304:dbl, "D"=w305:dbl, "V6d"=w290:dbl, "V0d"=w289:dbl, "C2V"=w287:u16, "V2C"=w288:u16)
                    n153 = Equal To 0?(x=w287) -> (x = 0?=w285:bool)
                    n154 = Equal To 0?(x=w288) -> (x = 0?=w286:bool)
                    n155 = call "Calculate V2C.vi"("Tcal_Chamber"=w309, "Voltage In"=w290, "Calibration Coefficients"=w292) -> ("C'"=w294:dbl, "B'"=w295:dbl, "A'"=w296:dbl, "CO2 Out"=w291:dbl, "D'"=w293:dbl)  [unwired: 4 in]
                    n156 = call "Calculate V2C.vi"("Tcal_Chamber"=w309, "Voltage In"=w289, "Calibration Coefficients"=w292) -> ("C'"=w300:dbl, "B'"=w301:dbl, "A'"=w302:dbl, "CO2 Out"=w297:dbl, "D'"=w299:dbl)  [unwired: 4 in]
                    n157 = Not And(1:w286, 2:w285) -> (0:w284:bool)
                    n158 = Subtract(x=w290, y=w289) -> (x-y=w283:dbl)
                    n159 = Less Than 0?(x=w283) -> (x < 0?=w282:bool)
                    n160 = Bundle By Name(cluster=w292, "C6d"=w291, "A'"=w296, "B'"=w295, "C'"=w294, "D'"=w293, "C0d"=w297) -> (w306:T2)
                  }
                  "V_0d(target)" <- w265
                  "V_6d(target)" <- w266
                  "V_span(target)" <- w277
                  "C6FC2V" <- w267
                  "A" <- w273
                  "B" <- w274
                  "C" <- w275
                  "D" <- w276
                  "B'" <- w270
                  "C'" <- w271
                  "D'" <- w272
                  "A'" <- w269
                  "C0FC2V" <- w268
                  "Status" <- w263
                  "BlueLED" <- w262
                  "BlueLED 2" <- w262
                  n161 = Increment(x=w281) -> (x+1=w278:u8)
                  n162 = local write "Coefficients_Out"(w279) -> ()
                }
                frame 2, Default {
                  n163 = Greater?(x=w320, y=u8 50) -> (0:w313:bool)
                  n164 = Increment(x=w318) -> (x+1=w316:T4)
                  n165 = Select(t=w316, s=w313, f=w318) -> (s? t:f=w317:T4)
                  n166 = Not(x=w313) -> (.not. x?=w311:bool)
                  n167 = local read "Cal Fail"() -> (w310:bool)
                  n168 = Increment(x=w320) -> (x+1=w315:u8)
                  n169 = Select(t=w315, s=w311, f=u8 0) -> (s? t:f=w312:u8)
                  n170 = property on="Cal Fail" class="Bool (strict)"("Visible"=w310, "Blinking"=w310) -> ()  [unwired: 2 in, 2 out]
                }
              }
            }
            frame "Setting Zero Point" {
              w330 = 4 ("index")
              # "ZERO COMPLETE - MOVE TO NEXT SEQUENCE"
              n171 = Build Array(w334) -> (→"Zero":dbl[][])
              n172 = local read "I_span"() -> (w326:dbl[])
              n173 = Initialize Array(0.015, w330) -> (w329:dbl[])
              n174 = Initialize Array(0.005, w330) -> (w328:dbl[])
              n175 = local read "Status"() -> (w325:bool[])
              n176 = case shown="9" w324 {
                selector: w324 -> [_ w362 w373 w378 w399 w428 w434 w445 w450 w466 w503 w523 w533 w557 w562 _]
                tunnel: [1 w361 w371 w376 w398 w427 w433 w443 w448 w465 w504 w522 w532 w556 w561 0] -> w338
                tunnel: w344 -> [w353 w360 w370 w377 w400 w426 w432 w442 w449 w473 w506 w524 w531 w558 w563 w568]
                tunnel: [w353 w360 w370 w377 w400 w426 w432 w442 w449 w473 w506 w524 w531 w558 w563 w567] -> w343
                tunnel: 20 ("y") -> [_ _ w367 _ _ _ _ w439 _ _ _ _ _ _ _ _]
                tunnel: w337 -> [_ _ _ w375 w394 w422 w430 w436 w447 w472 w505 w525 w535 w552 w564 w566]
                tunnel: w336 -> [w349 w358 w366 _ _ _ _ _ _ _ _ _ _ _ _ _]
                tunnel: 5 ("index") -> [_ _ _ _ _ _ _ _ _ _ _ _ _ _ _ _]
                tunnel: u8 0 ("CalGasTank") -> [w351 _ _ _ _ w424 _ _ _ _ _ _ _ _ _ _]
                tunnel: w328 -> [w346 w354 w363 w374 w388 _ _ _ _ _ w501 _ _ _ _ _]
                tunnel: w329 -> [_ _ _ _ _ w421 w429 w435 w446 w460 w502 _ _ _ _ _]
                tunnel: [w349 w358 w366 w375 w394 w422 w430 w436 w447 w472 w505 w525 w535 w552 w564 w566] -> w335
                tunnel: w334 -> [_ _ _ _ w392 _ _ _ _ w464 _ _ _ _ _ _]
                tunnel: [w346 w354 w363 w374 w388 w421 w429 w435 w446 w460 w494 w520 w530 w559 w560 w565] -> w327
                tunnel: w326 -> [_ _ _ _ _ _ _ _ _ _ w494 w520 w530 w559 w560 w565]
                tunnel: w325 -> [_ _ _ _ w379 _ _ _ _ w451 w493 _ _ _ _ _]
                frame 0 {
                  w345 = FALSE ("Visible")
                  # "SET DAC AND GAS TANK"
                  n177 = local write "CalGasTank"(w351) -> ()
                  n178 = local write "SetDac"(TRUE ("InCal")) -> ()
                  n179 = Not(x=w345) -> (.not. x?=w347:bool)
                  n180 = property on="Zero" class="WFChart (strict)"("Visible"=w347) -> ()  [unwired: 2 in, 2 out]
                  n181 = property on="mI" class="Arr (strict)"("Visible"=w345) -> ()  [unwired: 2 in, 2 out]
                  n182 = property on="V_RA(5mA)" class="Arr (strict)"("Visible"=w345) -> ()  [unwired: 2 in, 2 out]
                  n183 = property on="V_RA(15mA)" class="Arr (strict)"("Visible"=w345) -> ()  [unwired: 2 in, 2 out]
                  n184 = property on="DAC scale" class="Arr (strict)"("Visible"=w345) -> ()  [unwired: 2 in, 2 out]
                  n185 = property on="BlueLED" class="Arr (strict)"("Visible"=w345) -> ()  [unwired: 2 in, 2 out]
                  n186 = property on="CHANNEL 2" class="Arr (strict)"("Visible"=w345) -> ()  [unwired: 2 in, 2 out]
                  "Zero Status" <- T7."Setting Zero at 5 mA" ("Zero Status")
                }
                frame 1 {
                  # "CLEAR HISTORY WRITE DAC"
                  n187 = property on="Zero" class="WFChart (strict)"("History Data"=dbl[][] []) -> ()  [unwired: 2 in, 2 out]
                  n188 = Initialize Array(0, 4 ("dimension size")) -> (w356:i32[])
                  n189 = local write "mI"(w356) -> ()
                  n190 = local write "V_RA(15mA)"(w356) -> ()
                  n191 = local write "V_RA(5mA)"(w356) -> ()
                  n192 = Increment(x=w362) -> (x+1=w361:u8)
                }
                frame 2 {
                  # "WAIT FOR FIRST1 SECS"
                  n193 = property on="Zero" class="WFChart (strict)"() -> ("History Data"=w368:dbl[][])  [unwired: 2 in, 2 out]
                  n194 = Array Size(array=w368) -> (size(s)=w365:i32[])
                  n195 = Add Array Elements(numeric array=w365) -> (sum=w364:i32)
                  n196 = Greater?(x=w364, y=w367) -> (0:w369:bool)
                  n197 = Increment(x=w373) -> (x+1=w372:u8)
                  n198 = Select(t=w372, s=w369, f=w373) -> (s? t:f=w371:u8)
                }
                frame 3 {
                  # "IGNORE FIRST1 SECS - RESET AIRFLOW"
                  n199 = Increment(x=w378) -> (x+1=w376:u8)
                }
                frame 4 {
                  # "RUN TEST UNTIL STABLE"
                  n200 = property on="Zero" class="WFChart (strict)"() -> ("History Data"=w390:dbl[][])  [unwired: 2 in, 2 out]
                  n201 = Transpose 2D Array(2D array=w390) -> (transposed array=w389:dbl[][])
                  n202 = for {
                    tunnel: w389 -> [w407] mode=indexing
                    tunnel: w392 -> [w406] mode=indexing
                    tunnel: [w405] -> w387 mode=indexing
                    tunnel: [w404] -> w391 mode=indexing
                    tunnel: [w403] -> w380 mode=indexing
                    tunnel: w379 -> [w402] mode=indexing
                    n203 = case shown="True" w402 {
                      tunnel: w407 -> [_ w415]
                      tunnel: w406 -> [_ w414]
                      tunnel: [TRUE w413] -> w405
                      tunnel: [0.0 ("mean") w412] -> w404
                      tunnel: [0.0 w411] -> w403
                      frame False {
                      }
                      frame True {
                        n204 = Reverse 1D Array(array=w415) -> (reversed array=w416:dbl[])
                        n205 = Split 1D Array(array=w416, index=16) -> (first subarray=w417:dbl[])  [unwired: 1 out]
                        n206 = call-poly <vilib>:"Mean.vi"("X"=w417) -> ("mean"=w412:dbl)  [unwired: 1 out]
                        n207 = Subtract(x=w412, y=w414) -> (x-y=w419:dbl)
                        n208 = Absolute Value(x=w419) -> (abs(x)=w411:dbl)
                        n209 = Less Or Equal?(x=w411, y=0.001) -> (x <= y?=w413:bool)
                      }
                    }
                  }
                  "V_RA(5mA)" <- w391
                  n210 = Array Size(array=w389) -> (size(s)=w397:i32[])
                  n211 = Add Array Elements(numeric array=w397) -> (sum=w382:i32)
                  n212 = Greater?(x=w382, y=40 ("index")) -> (0:w395:bool)
                  n213 = Greater?(x=w382, y=100 ("index")) -> (0:w383:bool)
                  n214 = Increment(x=w399) -> (x+1=w401:u8)
                  n215 = Add Array Elements(numeric array=w380) -> (sum=w381:dbl)
                  n216 = And Array Elements(Boolean array=w387) -> (logical AND=w386:bool)
                  n217 = And(x=w395, y=w386) -> (x .and. y?=w384:bool)
                  n218 = Compound Arithmetic op=OR(w383, w384) -> (w393:bool)
                  n219 = Select(t=w401, s=w393, f=w399) -> (s? t:f=w398:u8)
                  n220 = local write "delta 2"(w381) -> ()
                }
                frame 5 {
                  # "SET DAC AND GAS TANK"
                  n221 = local write "CalGasTank"(w424) -> ()
                  n222 = local write "SetDac"(TRUE ("InCal")) -> ()
                  n223 = local write "Zero Status"(T7."Setting Zero at 15 mA" ("Zero Status")) -> ()
                  n224 = Increment(x=w428) -> (x+1=w427:u8)
                }
                frame 6 {
                  # "CLEAR HISTORY WRITE DAC"
                  n225 = property on="Zero" class="WFChart (strict)"("History Data"=dbl[][] []) -> ()  [unwired: 2 in, 2 out]
                  n226 = Increment(x=w434) -> (x+1=w433:u8)
                }
                frame 7 {
                  # "WAIT FOR FIRST 1 SECS"
                  n227 = property on="Zero" class="WFChart (strict)"() -> ("History Data"=w440:dbl[][])  [unwired: 2 in, 2 out]
                  n228 = Array Size(array=w440) -> (size(s)=w441:i32[])
                  n229 = Add Array Elements(numeric array=w441) -> (sum=w438:i32)
                  n230 = Greater?(x=w438, y=w439) -> (0:w437:bool)
                  n231 = Increment(x=w445) -> (x+1=w444:u8)
                  n232 = Select(t=w444, s=w437, f=w445) -> (s? t:f=w443:u8)
                }
                frame 8 {
                  # "IGNORE FIRST 1 SECS - RESET AIRFLOW"
                  n233 = Increment(x=w450) -> (x+1=w448:u8)
                }
                frame 9 {
                  # "RUN TEST UNTIL STABLE"
                  n234 = property on="Zero" class="WFChart (strict)"() -> ("History Data"=w462:dbl[][])  [unwired: 2 in, 2 out]
                  n235 = Transpose 2D Array(2D array=w462) -> (transposed array=w461:dbl[][])
                  n236 = for {
                    tunnel: w461 -> [w479] mode=indexing
                    tunnel: w464 -> [w478] mode=indexing
                    tunnel: [w477] -> w459 mode=indexing
                    tunnel: [w476] -> w463 mode=indexing
                    tunnel: [w475] -> w452 mode=indexing
                    tunnel: w451 -> [w474] mode=indexing
                    n237 = case shown="True" w474 {
                      tunnel: w479 -> [_ w487]
                      tunnel: w478 -> [_ w486]
                      tunnel: [TRUE w485] -> w477
                      tunnel: [0.0 ("mean") w484] -> w476
                      tunnel: [0.0 w483] -> w475
                      frame False {
                      }
                      frame True {
                        n238 = Reverse 1D Array(array=w487) -> (reversed array=w488:dbl[])
                        n239 = Split 1D Array(array=w488, index=16) -> (first subarray=w489:dbl[])  [unwired: 1 out]
                        n240 = call-poly <vilib>:"Mean.vi"("X"=w489) -> ("mean"=w484:dbl)  [unwired: 1 out]
                        n241 = Subtract(x=w484, y=w486) -> (x-y=w491:dbl)
                        n242 = Absolute Value(x=w491) -> (abs(x)=w483:dbl)
                        n243 = Less Or Equal?(x=w483, y=0.001) -> (x <= y?=w485:bool)
                      }
                    }
                  }
                  "V_RA(15mA)" <- w463
                  n244 = Array Size(array=w461) -> (size(s)=w470:i32[])
                  n245 = Add Array Elements(numeric array=w470) -> (sum=w455:i32)
                  n246 = Greater?(x=w455, y=40 ("index")) -> (0:w468:bool)
                  n247 = Greater?(x=w455, y=100 ("index")) -> (0:w454:bool)
                  n248 = Increment(x=w466) -> (x+1=w471:u8)
                  n249 = Add Array Elements(numeric array=w452) -> (sum=→"delta 2":dbl)
                  n250 = And Array Elements(Boolean array=w459) -> (logical AND=w458:bool)
                  n251 = And(x=w468, y=w458) -> (x .and. y?=w457:bool)
                  n252 = Compound Arithmetic op=OR(w454, w457) -> (w467:bool)
                  n253 = Select(t=w471, s=w467, f=w466) -> (s? t:f=w465:u8)
                }
                frame 10 {
                  # "CALCULATE"
                  n254 = local read "V_RA(15mA)"() -> (w498:dbl[])
                  n255 = local read "V_RA(5mA)"() -> (w499:dbl[])
                  n256 = Subtract(x=w502, y=w501) -> (x-y=w500:dbl[])
                  n257 = for {
                    tunnel: w500 -> [w510] mode=indexing
                    tunnel: w499 -> [w511] mode=indexing
                    tunnel: w498 -> [w512] mode=indexing
                    tunnel: [w509] -> w497 mode=indexing
                    tunnel: [0.0 ("x*y")] -> w495 mode=indexing
                    tunnel: w493 -> [w507] mode=indexing
                    n258 = case shown="True" w507 {
                      tunnel: w512 -> [_ w518]
                      tunnel: w511 -> [_ w517]
                      tunnel: w510 -> [_ w515]
                      tunnel: [0.0 w514] -> w509
                      frame False {
                      }
                      frame True {
                        n259 = Subtract(x=w518, y=w517) -> (x-y=w516:dbl)
                        n260 = Divide(x=w516, y=w515) -> (x/y=w514:dbl)
                      }
                    }
                  }
                  "mI" <- w497
                  "I_delta" <- w495
                  n261 = local write "Zero Status"(T7."Calculating slopes" ("Zero Status")) -> ()
                  n262 = Increment(x=w503) -> (x+1=w504:u8)
                }
                frame 11 {
                  w519 = TRUE ("Visible")
                  # "ZERO COMPLETE - Display and wait one sec"
                  n263 = Not(x=w519) -> (.not. x?=w521:bool)
                  n264 = property on="Zero" class="WFChart (strict)"("Visible"=w521) -> ()  [unwired: 2 in, 2 out]
                  n265 = property on="mI" class="Arr (strict)"("Visible"=w519) -> ()  [unwired: 2 in, 2 out]
                  n266 = property on="V_RA(5mA)" class="Arr (strict)"("Visible"=w519) -> ()  [unwired: 2 in, 2 out]
                  n267 = property on="V_RA(15mA)" class="Arr (strict)"("Visible"=w519) -> ()  [unwired: 2 in, 2 out]
                  n268 = property on="DAC scale" class="Arr (strict)"("Visible"=w519) -> ()  [unwired: 2 in, 2 out]
                  n269 = Increment(x=w523) -> (x+1=w522:u8)
                  n270 = property on="BlueLED" class="Arr (strict)"("Visible"=w519) -> ()  [unwired: 2 in, 2 out]
                  n271 = property on="CHANNEL 2" class="Arr (strict)"("Visible"=w519) -> ()  [unwired: 2 in, 2 out]
                }
                frame 12 {
                  n272 = local read "Coefficients_In"() -> (w539:T2[])
                  n273 = local read "V_RA(5mA)"() -> (w537:dbl[])
                  n274 = local read "mI"() -> (w540:dbl[])
                  n275 = local read "V_RA(15mA)"() -> (w536:dbl[])
                  n276 = local write "OK 9"(FALSE) -> ()
                  n277 = local read "BlueLED"() -> (w526:bool[])
                  n278 = for {
                    tunnel: w540 -> [w544] mode=indexing
                    tunnel: w539 -> [w551] mode=indexing
                    tunnel: [w550] -> w538 mode=indexing
                    tunnel: w537 -> [w549] mode=indexing
                    tunnel: w536 -> [w548] mode=indexing
                    tunnel: [0.0] -> w529 mode=indexing
                    tunnel: [i8 0 ("Step")] -> w534 mode=indexing
                    tunnel: [w543] -> w528 mode=indexing
                    tunnel: [w542] -> w527 mode=indexing
                    tunnel: w526 -> [w542] mode=indexing
                    n279 = Bundle By Name(cluster=w551, "V_(RA,5mA)"=w549, "V_(RA,15mA)"=w548, "mI"=w544) -> (w550:T2)
                    n280 = Divide(x=50, y=w544) -> (x/y=w543:dbl)
                  }
                  "DAC scale" <- w528
                  "I'mBlue" <- w527
                  n281 = local write "Coefficients_Out"(w538) -> ()
                  n282 = local write "Step"(w534) -> ()
                  n283 = local write "I_delta"(w529) -> ()
                  n284 = Increment(x=w533) -> (x+1=w532:u8)
                }
                frame 13 {
                  # "Set DAC to start calgas early"
                  n285 = local read "Gas Tank"() -> (w555:u8)
                  n286 = local read "I_span"() -> (w554:dbl[])
                  n287 = local write "SetDac"(TRUE ("InCal")) -> ()
                  n288 = local write "DAC Currents"(w554) -> ()
                  n289 = local write "CalGasTank"(w555) -> ()
                  n290 = Increment(x=w557) -> (x+1=w556:u8)
                }
                frame 14, Default {
                  # "ZERO COMPLETE - Display and wait one sec"
                  n291 = Increment(x=w562) -> (x+1=w561:u8)
                }
                frame 30 {
                  n292 = Increment(x=w568) -> (x+1=w567:T4)
                }
              }
              n293 = local read "stage 2 - zeroing"() -> (w323:i16[][])
              n294 = local write "DAC Currents"(w327) -> ()
              n295 = local read "Index"() -> (w321:u16)
            }
            frame "Setting Span Point" {
              n296 = local read "V_span(target)"() -> (w579:dbl[])
              n297 = local read "V_span(ImA)"() -> (w578:dbl[])
              n298 = local read "V_0d(ImA)"() -> (w581:dbl[])
              n299 = local read "DAC scale"() -> (w575:dbl[])
              n300 = local read "I'mBlue"() -> (w576:bool[])
              n301 = Build Array(w582) -> (→"Span Point Calibration":dbl[][])
              n302 = local read "Status"() -> (w577:bool[])
              n303 = local read "DAC"() -> (w574:u16[])
              n304 = case shown="5" w573 {
                selector: w573 -> [w604 w621 w633 w635 w657 w696 w725 w736 w790 w822 w864 w868 w872 w876 w880 _]
                tunnel: "OK 9" -> [_ _ _ _ _ w692 _ _ _ w821 _ _ _ _ _ _]
                tunnel: [w603 w624 w632 w634 w658 w697 w724 w734 w789 w823 w863 w867 w871 w875 w879 0 ("Step")] -> w587
                tunnel: w592 -> [w606 w628 w631 w643 w660 w700 w723 w735 w788 w827 w861 w865 w869 w873 w877 w883]
                tunnel: [w606 w628 w631 w643 w660 w700 w723 w735 w788 w827 w861 w865 w869 w873 w877 w881] -> w591
                tunnel: w585 -> [w605 w620 w629 _ _ _ _ _ _ _ _ _ _ _ _ _]
                tunnel: w586 -> [_ _ _ w642 w654 w690 w722 w726 w787 w812 w862 w866 w870 w874 w878 w884]
                tunnel: w579 -> [_ _ _ _ w644 _ _ w733 w782 w820 _ _ _ _ _ _]
                tunnel: "Gas Tank" -> [w601 _ _ _ _ _ _ _ _ _ _ _ _ _ _ _]
                tunnel: [w605 w620 w629 w642 w654 w690 w722 w726 w787 w812 w862 w866 w870 w874 w878 w884] -> w584
                tunnel: w582 -> [_ _ _ _ w651 w689 _ _ _ _ _ _ _ _ _ _]
                tunnel: w581 -> [_ _ _ _ w650 w685 _ _ w778 _ _ _ _ _ _ _]
                tunnel: w578 -> [_ _ _ _ _ _ _ w730 w781 w819 _ _ _ _ _ _]
                tunnel: w577 -> [w594 _ _ _ w645 w680 _ w729 w780 w810 _ _ _ _ _ _]
                tunnel: w576 -> [_ _ _ _ _ _ _ w728 _ _ _ _ _ _ _ _]
                tunnel: w575 -> [_ _ _ _ _ _ _ w727 _ _ _ _ _ _ _ _]
                tunnel: w574 -> [_ _ _ _ _ _ _ _ w779 w811 _ _ _ _ _ _]
                frame 0, Default {
                  # "SET DAC AND GAS TANK"
                  n305 = local read "I_delta"() -> (w597:dbl[])
                  n306 = local read "I_span"() -> (w598:dbl[])
                  n307 = local read "mI"() -> (w600:dbl[])
                  n308 = local write "CalGasTank"(w601) -> ()
                  n309 = for {
                    tunnel: w600 -> [w610] mode=indexing
                    tunnel: [w609] -> w599 mode=indexing
                    tunnel: w598 -> [w612] mode=indexing
                    tunnel: w597 -> [w611] mode=indexing
                    tunnel: [w608] -> w596 mode=indexing
                    tunnel: [w608] -> w595 mode=indexing
                    tunnel: w594 -> [w607] mode=indexing
                    n310 = case shown="True" w607 {
                      tunnel: w612 -> [_ w618]
                      tunnel: w611 -> [_ w617]
                      tunnel: w610 -> [_ w616]
                      tunnel: [w613 w615] -> w609
                      tunnel: [w613 w614] -> w608
                      frame False {
                        w613 = 0.0
                      }
                      frame True {
                        n311 = Add(x=w618, y=w617) -> (x+y=w614:dbl)
                        n312 = Multiply(x=w614, y=w616) -> (x*y=w615:dbl)
                      }
                    }
                  }
                  "V_0d(ImA)" <- w599
                  n313 = Increment(x=w604) -> (x+1=w603:u8)
                  n314 = property on="Span Point Calibration" class="WFChart (strict)"("History Data"=dbl[][] []) -> ()  [unwired: 2 in, 2 out]
                  n315 = local write "DAC Currents"(w596) -> ()
                  n316 = local write "I_span"(w595) -> ()
                  n317 = local write "SetDac"(TRUE ("InCal")) -> ()
                }
                frame 1 {
                  # "Wait half a sec"
                  n318 = property on="Span Point Calibration" class="WFChart (strict)"() -> ("History Data"=w627:dbl[][])  [unwired: 2 in, 2 out]
                  n319 = Array Size(array=w627) -> (size(s)=w626:i32[])
                  n320 = Add Array Elements(numeric array=w626) -> (sum=w619:i32)
                  n321 = Greater?(x=w619, y=10) -> (0:w622:bool)
                  n322 = Increment(x=w621) -> (x+1=w623:u8)
                  n323 = Select(t=w623, s=w622, f=w621) -> (s? t:f=w624:u8)
                }
                frame 2 {
                  # "CLEAR HISTORY WRITE DAC"
                  # "Discard dac settling data"
                  n324 = property on="Span Point Calibration" class="WFChart (strict)"("History Data"=dbl[][] []) -> ()  [unwired: 2 in, 2 out]
                  n325 = Increment(x=w633) -> (x+1=w632:u8)
                }
                frame 3 {
                  # "Now accumulate one sec of data into buffer for mean calculation"
                  n326 = property on="Span Point Calibration" class="WFChart (strict)"() -> ("History Data"=w641:dbl[][])  [unwired: 2 in, 2 out]
                  n327 = Array Size(array=w641) -> (size(s)=w640:i32[])
                  n328 = Add Array Elements(numeric array=w640) -> (sum=w636:i32)
                  n329 = Greater?(x=w636, y=20) -> (0:w637:bool)
                  n330 = Increment(x=w635) -> (x+1=w638:u8)
                  n331 = Select(t=w638, s=w637, f=w635) -> (s? t:f=w634:u8)
                }
                frame 4 {
                  # "QUICK CHECK"
                  # "QUICK CHECK - that mean is within 1V of target - if any are not readjust and re-loop"
                  n332 = property on="Span Point Calibration" class="WFChart (strict)"() -> ("History Data"=w647:dbl[][])  [unwired: 2 in, 2 out]
                  n333 = Transpose 2D Array(2D array=w647) -> (transposed array=w646:dbl[][])
                  n334 = for {
                    tunnel: w646 -> [w666] mode=indexing
                    tunnel: [w668] -> w649 mode=indexing
                    tunnel: w651 -> [w667] mode=indexing
                    tunnel: [w664] -> w652 mode=indexing
                    tunnel: [w665] -> w653 mode=indexing
                    tunnel: w650 -> [w663] mode=indexing
                    tunnel: w645 -> [w662] mode=indexing
                    tunnel: w644 -> [w661] mode=indexing
                    n335 = case shown="True" w662 {
                      tunnel: [FALSE w679] -> w668
                      tunnel: w667 -> [_ _]
                      tunnel: w666 -> [_ w678]
                      tunnel: [w670 w677] -> w665
                      tunnel: [w670 w671] -> w664
                      tunnel: w663 -> [_ w676]
                      tunnel: w661 -> [_ w672]
                      frame False {
                        w670 = 0.0
                      }
                      frame True {
                        n336 = call-poly <vilib>:"Mean.vi"("X"=w678) -> ("mean"=w677:dbl)  [unwired: 1 out]
                        n337 = Subtract(x=w677, y=w676) -> (x-y=w671:dbl)
                        n338 = Subtract(x=w671, y=w672) -> (x-y=w673:dbl)
                        n339 = Absolute Value(x=w673) -> (abs(x)=w674:dbl)
                        n340 = Less Or Equal?(x=w674, y=1.0) -> (x <= y?=w679:bool)
                      }
                    }
                  }
                  n341 = Add(x=w657, y=2) -> (x+y=w655:i32)
                  n342 = local write "V_span(ImA)"(w652) -> ()
                  n343 = Or Array Elements(Boolean array=w649) -> (logical OR=w648:bool)
                  n344 = Increment(x=w657) -> (x+1=w659:u8)
                  n345 = local write "V_6d(ImA)"(w653) -> ()
                  n346 = Select(t=w659, s=w648, f=w655) -> (s? t:f=w658:i32)
                }
                frame 5 {
                  # "RUN TEST UNTIL STABLE"
                  # "We are within a volt for all channels so now check for stable signals"
                  n347 = property on="Span Point Calibration" class="WFChart (strict)"() -> ("History Data"=w684:dbl[][])  [unwired: 2 in, 2 out]
                  n348 = Transpose 2D Array(2D array=w684) -> (transposed array=w683:dbl[][])
                  n349 = for {
                    tunnel: w683 -> [w707] mode=indexing
                    tunnel: [w706] -> w682 mode=indexing
                    tunnel: w689 -> [w705] mode=indexing
                    tunnel: [w704] -> w688 mode=indexing
                    tunnel: [w703] -> w686 mode=indexing
                    tunnel: w685 -> [w702] mode=indexing
                    tunnel: w680 -> [w701] mode=indexing
                    n350 = case shown="True" w701 {
                      tunnel: w707 -> [_ w715]
                      tunnel: [FALSE w714] -> w706
                      tunnel: w705 -> [_ w713]
                      tunnel: [w709 w712] -> w704
                      tunnel: [w709 w710] -> w703
                      tunnel: w702 -> [_ w711]
                      frame False {
                        w709 = 0.0 ("mean")
                      }
                      frame True {
                        n351 = Reverse 1D Array(array=w715) -> (reversed array=w716:dbl[])
                        n352 = Split 1D Array(array=w716, index=16) -> (first subarray=w717:dbl[])  [unwired: 1 out]
                        n353 = call-poly <vilib>:"Mean.vi"("X"=w717) -> ("mean"=w710:dbl)  [unwired: 1 out]
                        n354 = Subtract(x=w710, y=w713) -> (x-y=w719:dbl)
                        n355 = Subtract(x=w710, y=w711) -> (x-y=w712:dbl)
                        n356 = Absolute Value(x=w719) -> (abs(x)=w720:dbl)
                        n357 = Less Or Equal?(x=w720, y=0.005) -> (x <= y?=w714:bool)
                      }
                    }
                  }
                  "V_span(ImA)" <- w688
                  "V_6d(ImA)" <- w686
                  n358 = Array Size(array=w683) -> (size(s)=w694:i32[])
                  n359 = Add Array Elements(numeric array=w694) -> (sum=w687:i32)
                  n360 = Greater?(x=w687, y=100 ("index")) -> (0:w693:bool)
                  n361 = Or(x=w692, y=w693) -> (x .or. y?=w691:bool)
                  n362 = Or Array Elements(Boolean array=w682) -> (logical OR=w681:bool)
                  n363 = Or(x=w691, y=w681) -> (x .or. y?=w698:bool)
                  n364 = Increment(x=w696) -> (x+1=w699:u8)
                  n365 = Select(t=w699, s=w698, f=w696) -> (s? t:f=w697:u8)
                }
                frame 6 {
                  n366 = Increment(x=w725) -> (x+1=w724:u8)
                }
                frame 7 {
                  # "CALCULATE"
                  n367 = for {
                    tunnel: w733 -> [w741] mode=indexing
                    tunnel: [w743] -> w732 mode=indexing
                    tunnel: [w742] -> w731 mode=indexing
                    tunnel: w730 -> [w740] mode=indexing
                    tunnel: w729 -> [w739] mode=indexing
                    tunnel: w728 -> [w738] mode=indexing
                    tunnel: w727 -> [w737] mode=indexing
                    n368 = case shown="True" w739 {
                      tunnel: [0.0 w765] -> w743
                      tunnel: [i8 0 ("t") w746] -> w742
                      tunnel: w741 -> [_ w764]
                      tunnel: w740 -> [_ w763]
                      tunnel: w738 -> [_ w759]
                      tunnel: w737 -> [_ w758]
                      frame False {
                      }
                      frame True {
                        # "Scale DAC"
                        n369 = Subtract(x=w764, y=w763) -> (x-y=w770:dbl)
                        n370 = Absolute Value(x=w770) -> (abs(x)=w751:dbl)
                        n371 = Less Than 0?(x=w770) -> (x < 0?=w756:bool)
                        n372 = Less Or Equal?(x=w751, y=0.1) -> (x <= y?=w776:bool)
                        n373 = Less Or Equal?(x=w751, y=0.25) -> (x <= y?=w771:bool)
                        n374 = Less Or Equal?(x=w751, y=0.5) -> (x <= y?=w750:bool)
                        n375 = Less Or Equal?(x=w751, y=1.0) -> (x <= y?=w752:bool)
                        n376 = Select(t=i8 1, s=w776, f=i8 3 ("t")) -> (s? t:f=w760:i8)
                        n377 = Select(t=w760, s=w771, f=i8 10 ("t")) -> (s? t:f=w767:i8)
                        n378 = Select(t=w767, s=w750, f=i8 30 ("t")) -> (s? t:f=w749:i8)
                        n379 = Select(t=w749, s=w752, f=i8 60 ("t")) -> (s? t:f=w748:i8)
                        n380 = Not(x=w756) -> (.not. x?=w755:bool)
                        n381 = Multiply(x=w758, y=w748) -> (x*y=w757:dbl)
                        n382 = Select(t=w755, s=w759, f=w756) -> (s? t:f=w761:bool)
                        n383 = Negate(x=w757) -> (-x=w762:dbl)
                        n384 = Select(t=w762, s=w761, f=w757) -> (s? t:f=w747:dbl)
                        n385 = To Word Integer(number=w747) -> (16bit integer=w746:i16)
                        n386 = Multiply(x=0.0001 ("y"), y=w746) -> (x*y=w765:dbl)
                      }
                    }
                  }
                  "Step" <- w731
                  n387 = Increment(x=w736) -> (x+1=w734:u8)
                  n388 = local write "I_delta"(w732) -> ()
                }
                frame 8 {
                  # "Coarse update to approx CO2 calc"
                  n389 = local read "V_0d(target)"() -> (w783:dbl[])
                  n390 = local read "I_span"() -> (w784:dbl[])
                  n391 = local read "Coefficients_In"() -> (w786:T2[])
                  n392 = for {
                    tunnel: w786 -> [w800] mode=indexing
                    tunnel: [w799] -> w785 mode=indexing
                    tunnel: w779 -> [w798] mode=indexing
                    tunnel: w784 -> [w797] mode=indexing
                    tunnel: w778 -> [w796] mode=indexing
                    tunnel: w783 -> [w792] mode=indexing
                    tunnel: w782 -> [w795] mode=indexing
                    tunnel: w781 -> [w793] mode=indexing
                    tunnel: w780 -> [w794] mode=indexing
                    n393 = Add(x=w792, y=w793) -> (x+y=w791:dbl)
                    n394 = case shown="True" w794 {
                      tunnel: [w803 w809] -> w802
                      tunnel: [w803 w808] -> w801
                      tunnel: w796 -> [_ w807]
                      tunnel: w792 -> [_ w806]
                      tunnel: w795 -> [_ w805]
                      tunnel: w793 -> [_ w804]
                      frame False {
                        w803 = 0.0
                      }
                      frame True {
                        n395 = Subtract(x=w807, y=w806) -> (x-y=w808:dbl)
                        n396 = Divide(x=w805, y=w804) -> (x/y=w809:dbl)
                      }
                    }
                    n397 = Bundle By Name(cluster=w800, "V_6d_ImA (actual)"=w791, "DAC"=w798, "I_span"=w797, "V_offs"=w801, "G_adj"=w802) -> (w799:T2)
                  }
                  n398 = Increment(x=w790) -> (x+1=w789:u8)
                  n399 = local write "Coefficients_Out"(w785) -> ()
                }
                frame 9 {
                  # "CALCULATE"
                  n400 = local read "I_delta"() -> (w815:dbl[])
                  n401 = local read "Step"() -> (w818:i16[])
                  n402 = for {
                    tunnel: w820 -> [w842] mode=indexing
                    tunnel: w819 -> [w841] mode=indexing
                    tunnel: w818 -> [w840] mode=indexing
                    tunnel: [w836] -> w813 mode=indexing
                    tunnel: [w839] -> w816 mode=indexing
                    tunnel: w815 -> [w838] mode=indexing
                    tunnel: [w837] -> w814 mode=indexing
                    tunnel: w811 -> [w832] mode=indexing
                    tunnel: [w829] -> _ mode=indexing
                    tunnel: w810 -> [w829] mode=indexing
                    n403 = Equal To 0?(x=w832) -> (x = 0?=w835:bool)
                    n404 = Equal?(x=w832, y=u16 1023) -> (x = y?=w834:bool)
                    n405 = Or(x=w835, y=w834) -> (x .or. y?=w831:bool)
                    n406 = Not(x=w831) -> (.not. x?=w830:bool)
                    n407 = And(x=w830, y=w829) -> (x .and. y?=w828:bool)
                    n408 = case shown="True" w828 {
                      tunnel: w842 -> [_ w853]
                      tunnel: w841 -> [_ w852]
                      tunnel: w840 -> [_ w851]
                      tunnel: [i8 0 ("Step") w850] -> w839
                      tunnel: w838 -> [_ w849]
                      tunnel: [0.0 ("V_(RA,5mA)") w847] -> w837
                      tunnel: [TRUE w846] -> w836
                      frame False {
                      }
                      frame True {
                        w848 = i8 0 ("t")
                        n409 = Subtract(x=w853, y=w852) -> (x-y=w854:dbl)
                        n410 = Absolute Value(x=w854) -> (abs(x)=w855:dbl)
                        n411 = Less?(x=w855, y=0.05) -> (x < y?=w846:bool)
                        n412 = Select(t=w848, s=w846, f=w851) -> (s? t:f=w850:i16)
                        n413 = Select(t=w848, s=w846, f=w849) -> (s? t:f=w847:dbl)
                      }
                    }
                  }
                  n414 = And Array Elements(Boolean array=w813) -> (logical AND=w817:bool)
                  n415 = Or(x=w821, y=w817) -> (x .or. y?=w824:bool)
                  n416 = local write "Step"(w816) -> ()
                  n417 = local write "I_delta"(w814) -> ()
                  n418 = local write "Span Good"(w813) -> ()
                  n419 = Increment(x=w822) -> (x+1=w825:u8)
                  n420 = Select(t=w825, s=w824, f=0) -> (s? t:f=w823:i32)
                }
                frame 10 {
                  # "Just delay a few counts to allow storage of a few correct CO2s"
                  n421 = local write "CalGasTank"(u8 0 ("CalGasTank")) -> ()
                  n422 = local write "SetDac"(TRUE ("InCal")) -> ()
                  n423 = Increment(x=w864) -> (x+1=w863:u8)
                  n424 = local write "OK 10"(FALSE ("OK 10")) -> ()
                  n425 = property on="Zero Offset" class="WFChart (strict)"("History Data"=dbl[][] []) -> ()  [unwired: 2 in, 2 out]
                }
                frame 11 {
                  # "Just delay a few counts to allow storage of a few correct CO2s"
                  n426 = Increment(x=w868) -> (x+1=w867:u8)
                }
                frame 12 {
                  # "Just delay a few counts to allow storage of a few correct CO2s"
                  n427 = Increment(x=w872) -> (x+1=w871:u8)
                }
                frame 13 {
                  # "Just delay a few counts to allow storage of a few correct CO2s"
                  n428 = Increment(x=w876) -> (x+1=w875:u8)
                }
                frame 14 {
                  # "Just delay a few counts to allow storage of a few correct CO2s"
                  n429 = Increment(x=w880) -> (x+1=w879:u8)
                }
                frame 15 {
                  # "Now Exit"
                  n430 = Increment(x=w883) -> (x+1=w881:T4)
                }
              }
              n431 = Subtract(x=w579, y=w578) -> (x-y=w580:dbl[])
              n432 = local write "V_Span Delta"(w580) -> ()
              n433 = local read "stage 3 - span"() -> (w572:i16[][])
              n434 = local read "Index"() -> (w571:u16)
            }
            frame "Calculating Gain & Offset" {
              w895 = u16 450  # Fast AirPump
              n435 = Build Array(w891) -> (→"Zero Offset":dbl[][])
              n436 = local read "Status"() -> (w889:bool[])
              n437 = case shown="5" w887 {
                selector: w887 -> [_ w907 w917 w921 w931 w961 _]
                tunnel: [1 w906 w915 w919 w930 w965 1] -> w897
                tunnel: w899 -> [w903 w905 w914 w920 w932 w966 w988]
                tunnel: [w903 w905 w914 w920 w932 w966 w987] -> w898
                tunnel: w894 -> [_ _ _ w918 w923 _ _]
                tunnel: w895 -> [w901 w904 w909 _ _ _ _]
                tunnel: [w901 w904 w909 w918 w923 w957 w985] -> w896
                tunnel: w893 -> [_ _ _ _ _ w957 w985]
                tunnel: w891 -> [_ _ _ _ w926 _ _]
                tunnel: w889 -> [_ _ _ _ w922 w949 _]
                frame 0, Default {
                  # "SET DAC AND GAS TANK\n\nMOVED TO END OF SPAN TO SHOW FINAL NUMBERS"
                }
                frame 1 {
                  # "CLEAR HISTORY WRITE DAC"
                  n438 = Increment(x=w907) -> (x+1=w906:u8)
                }
                frame 2 {
                  # "WAIT FOR FIRST 5 SECS"
                  n439 = property on="Zero Offset" class="WFChart (strict)"() -> ("History Data"=w911:dbl[][])  [unwired: 2 in, 2 out]
                  n440 = Array Size(array=w911) -> (size(s)=w913:i32[])
                  n441 = Add Array Elements(numeric array=w913) -> (sum=w908:i32)
                  n442 = Greater?(x=w908, y=40) -> (0:w912:bool)
                  n443 = Increment(x=w917) -> (x+1=w916:u8)
                  n444 = Select(t=w916, s=w912, f=w917) -> (s? t:f=w915:u8)
                }
                frame 3 {
                  # "IGNORE FIRST 2 SECS - RESET AIRFLOW"
                  n445 = Increment(x=w921) -> (x+1=w919:u8)
                }
                frame 4 {
                  # "RUN TEST UNTIL STABLE"
                  n446 = property on="Zero Offset" class="WFChart (strict)"() -> ("History Data"=w929:dbl[][])  [unwired: 2 in, 2 out]
                  n447 = Transpose 2D Array(2D array=w929) -> (transposed array=w928:dbl[][])
                  n448 = for {
                    tunnel: w928 -> [w937] mode=indexing
                    tunnel: [w936] -> w927 mode=indexing
                    tunnel: w926 -> [w935] mode=indexing
                    tunnel: [w934] -> w925 mode=indexing
                    tunnel: w922 -> [w933] mode=indexing
                    n449 = case shown="False" w933 {
                      tunnel: w937 -> [_ w942]
                      tunnel: [w938 w941] -> w936
                      tunnel: w935 -> [_ w940]
                      tunnel: [w938 w939] -> w934
                      frame False {
                        w938 = 0.0 ("mean")
                      }
                      frame True {
                        n450 = Reverse 1D Array(array=w942) -> (reversed array=w943:dbl[])
                        n451 = Split 1D Array(array=w943, index=16) -> (first subarray=w944:dbl[])  [unwired: 1 out]
                        n452 = call-poly <vilib>:"Mean.vi"("X"=w944) -> ("mean"=w941:dbl)  [unwired: 1 out]
                        n453 = Subtract(x=w941, y=w940) -> (x-y=w946:dbl)
                        n454 = Absolute Value(x=w946) -> (abs(x)=w939:dbl)
                      }
                    }
                  }
                  n455 = Increment(x=w931) -> (x+1=w930:u8)
                  n456 = Add Array Elements(numeric array=w925) -> (sum=→"delta":dbl)
                  n457 = local write "V_0d(ImA)"(w927) -> ()
                }
                frame 5 {
                  # "CALCULATE"
                  n458 = local read "V_span(target)"() -> (w951:dbl[])
                  n459 = local read "V_0d(target)"() -> (w952:dbl[])
                  n460 = local read "V_6d(ImA)"() -> (w950:dbl[])
                  n461 = local read "V_0d(ImA)"() -> (w953:dbl[])
                  n462 = for {
                    tunnel: [w975] -> w956 mode=indexing
                    tunnel: [w974] -> w955 mode=indexing
                    tunnel: [w973] -> w954 mode=indexing
                    tunnel: w953 -> [w972] mode=indexing
                    tunnel: w951 -> [w971] mode=indexing
                    tunnel: w952 -> [w970] mode=indexing
                    tunnel: w950 -> [w969] mode=indexing
                    tunnel: [w968] -> w948 mode=indexing
                    tunnel: w949 -> [w967] mode=indexing
                    n463 = case shown="True" w967 {
                      tunnel: [w976 w984] -> w975
                      tunnel: [w976 w983] -> w974
                      tunnel: [w976 w982] -> w973
                      tunnel: w972 -> [_ w981]
                      tunnel: w971 -> [_ w980]
                      tunnel: w970 -> [_ w979]
                      tunnel: w969 -> [_ w978]
                      tunnel: [w976 0.001] -> w968
                      frame False {
                        w976 = 0.0
                      }
                      frame True {
                        n464 = Subtract(x=w978, y=w981) -> (x-y=w983:dbl)
                        n465 = Subtract(x=w981, y=w979) -> (x-y=w982:dbl)
                        n466 = Divide(x=w980, y=w983) -> (x/y=w984:dbl)
                      }
                    }
                  }
                  "V_0(adjust)" <- w954
                  "V_span(adjust)" <- w955
                  "Gain(adjust)" <- w956
                  n467 = local read "delta"() -> (w964:dbl)
                  n468 = Increment(x=w961) -> (x+1=w963:u8)
                  n469 = Decrement(x=w961) -> (x-1=w962:u8)
                  n470 = Add Array Elements(numeric array=w948) -> (sum=w947:dbl)
                  n471 = Less Or Equal?(x=w964, y=w947) -> (x <= y?=w960:bool)
                  n472 = Or(x=w960, y="OK 10") -> (x .or. y?=w959:bool)
                  n473 = Select(t=w963, s=w959, f=w962) -> (s? t:f=w965:u8)
                }
                frame 6 {
                  # "GAIN & OFFSET COMPLETE - MOVE TO NEXT SEQUENCE"
                  n474 = call <vilib>:"Beep.vi"() -> ()  [unwired: 12 in]
                  n475 = Increment(x=w988) -> (x+1=w987:T4)
                }
              }
              n476 = property on="DAC Currents" class="Arr (strict)"("Visible"=TRUE) -> ()  [unwired: 2 in, 2 out]
              n477 = local read "stage 4 - offset adjust"() -> (w888:i16[][])
              n478 = local read "Index"() -> (w886:u16)
            }
            frame "Storing Calibration Coefficients" {
              w989 = 0
              n479 = case shown="1" w994 {
                selector: w994 -> [w1007 w1032 w1065 w1071]
                tunnel: w999 -> [w1011 w1030 w1063 w1076]
                tunnel: [w1006 w1030 w1063 w1075] -> w998
                tunnel: w997 -> [w1013 w1038 w1067 w1074]
                tunnel: [w1010 w1037 w1066 w1073] -> w996
                tunnel: w995 -> [w1012 w1026 w1062 w1069]
                tunnel: [w1007 w1031 w1064 w1070] -> w993
                tunnel: [w1012 w1026 w1062 w1069] -> w992
                tunnel: w991 -> [w1008 w1027 _ _]
                frame 0 {
                  w1005 = FALSE ("Visible")
                  # "This case is only reached when skip calibration is selected at the start"
                  n480 = local read "time_now"() -> (w1009:timestamp)
                  n481 = local read "Coefficients_In"() -> (w1002:T2[])
                  n482 = Subtract(x=w1009, y=w1008) -> (x-y=w1004:dbl)
                  n483 = for {
                    tunnel: w1004 -> [w1016]
                    tunnel: "CAL SKIPPED" -> [w1017]
                    tunnel: w1002 -> [w1015] mode=indexing
                    tunnel: [w1014] -> w1001 mode=indexing
                    n484 = Bundle By Name(cluster=w1015, "cal_utc"=w1016, "zero_utc"=w1016, "TYPE"=w1017) -> (w1014:T2)
                  }
                  n485 = local write "Coefficients_Out"(w1001) -> ()
                  n486 = local write "Quit"(TRUE ("Cal Fail")) -> ()
                  n487 = Decrement(x=w1013) -> (x-1=w1010:u16)
                  n488 = property on="elapsed time" class="DigNum (strict)"("Visible"=w1005) -> ()  [unwired: 2 in, 2 out]
                  n489 = Increment(x=w1011) -> (x+1=w1006:T4)
                  n490 = property on="Quit" class="Bool (strict)"("Visible"=w1005) -> ()  [unwired: 2 in, 2 out]
                }
                frame 1 {
                  w1023 = TRUE ("want seconds? (F)")
                  n491 = local read "elapsed time"() -> (w1033:i16)
                  "duration" <- w1033
                  n492 = local read "time_now"() -> (w1029:timestamp)
                  "Calibration Complete -" <- w1029
                  n493 = Subtract(x=w1029, y=w1027) -> (x-y=w1028:dbl)
                  n494 = local read "Coefficients_In"() -> (w1024:T2[])
                  n495 = local read "Gain(adjust)"() -> (w1020:dbl[])
                  n496 = local read "V_0(adjust)"() -> (w1021:dbl[])
                  n497 = local read "Status"() -> (w1018:bool[])
                  n498 = local read "V_6d(ImA)"() -> (w1019:dbl[])
                  n499 = local read "V_0d(ImA)"() -> (w1022:dbl[])
                  n500 = Get Date/Time String(date format (0)=enum16{"short", "long", "abbreviated"}."short", seconds (now)=w1029, want seconds? (F)=w1023) -> (date string=w1034:string, time string=w1035:string)
                  n501 = for {
                    tunnel: w1023 -> [_]
                    tunnel: w1035 -> [w1043]
                    tunnel: w1034 -> [w1045]
                    tunnel: w1033 -> [w1041]
                    tunnel: w1028 -> [w1047]
                    tunnel: w1026 -> [w1054]
                    tunnel: [w1053] -> w1025 mode=indexing
                    tunnel: w1024 -> [w1052] mode=indexing
                    tunnel: w1022 -> [w1039] mode=indexing
                    tunnel: w1021 -> [w1051] mode=indexing
                    tunnel: w1020 -> [w1050] mode=indexing
                    tunnel: w1019 -> [w1049] mode=indexing
                    tunnel: w1018 -> [w1048] mode=indexing
                    n502 = case shown="False" w1048 {
                      tunnel: [0.0 w1061] -> w1046
                      tunnel: w1047 -> [_ w1061]
                      tunnel: w1045 -> [_ w1060]
                      tunnel: [w1055 w1060] -> w1044
                      tunnel: w1043 -> [_ w1059]
                      tunnel: [w1055 w1059] -> w1042
                      tunnel: w1041 -> [_ w1058]
                      tunnel: [i16 0 ("elapsed time") w1058] -> w1040
                      frame False {
                        w1055 = ""
                      }
                      frame True {
                      }
                    }
                    n503 = Bundle By Name(cluster=w1052, "cal_utc"=w1046, "CalDate"=w1044, "CalTime"=w1042, "duration"=w1040, "V_(()d, average)"=w1039, "V_0d_ImA (actual)"=w1039, "V_6d_ImA (actual)"=w1049, "cal_offs_adj"=w1051, "cal_gain_adj"=w1050, "V_offs"=w1051, "G_adj"=w1050, "Pump Flow Rate"=w1054) -> (w1053:T2)
                  }
                  n504 = local write "Coefficients_Out"(w1025) -> ()
                  n505 = Increment(x=w1032) -> (x+1=w1031:u8)
                  n506 = Decrement(x=w1038) -> (x-1=w1037:u16)
                }
                frame 2, Default {
                  n507 = Increment(x=w1065) -> (x+1=w1064:u8)
                  n508 = Decrement(x=w1067) -> (x-1=w1066:u16)
                }
                frame 20 {
                  w1072 = FALSE ("Visible")
                  n509 = Decrement(x=w1074) -> (x-1=w1073:u16)
                  n510 = Increment(x=w1071) -> (x+1=w1070:u8)
                  n511 = property class="VI"("Exec.CloseFPAfterCall"=TRUE ("Execution:Close After Call")) -> ()  [unwired: 2 in, 2 out]
                  n512 = property on="elapsed time" class="DigNum (strict)"("Visible"=w1072) -> ()  [unwired: 2 in, 2 out]
                  n513 = property on="Quit" class="Bool (strict)"("Visible"=w1072) -> ()  [unwired: 2 in, 2 out]
                  n514 = Increment(x=w1076) -> (x+1=w1075:T4)
                }
              }
            }
            frame "Calibration Complete" {
              w1077 = 0 ("Count")
              w1079 = TRUE
              n515 = Decrement(x=w1083) -> (x-1=w1082:u16)
              n516 = property class="VI"("Exec.CloseFPAfterCall"=w1079) -> ()  [unwired: 2 in, 2 out]
              n517 = case shown="True" w1079 {
                frame False {
                }
                frame True {
                  n518 = local write "Quit"(FALSE) -> ()
                  n519 = property class="VI"("FP.State"=T8."Closed" ("Front Panel Window:State")) -> ()  [unwired: 2 in, 2 out]
                }
              }
              "Calibration Complete" <- w1079
            }
          }
          "Count" <- w48
          "Actual" <- w46
          n520 = call "Get Pump Sequence.vi"("Array"=w38, "Index"=w40, "Stage"=w41) -> ("Error"=→"Error":bool, "Pump Settings"=→"Pump Settings":T1, "Updated Index"=→"Index":u16, "Ignore"=w35:bool)  [unwired: 5 in]
          n521 = Not(x=w35) -> (.not. x?=w34:bool)
          n522 = property on="Pump Settings" class="Clust (strict)"("Visible"=w34) -> ()  [unwired: 2 in, 2 out]
        }
        frame True {
          w1087 = FALSE ("Calibration Complete")
          n523 = property class="VI"("Exec.CloseFPAfterCall"=w1087, "FP.State"=T8."Standard" ("Front Panel Window:State")) -> ()  [unwired: 2 in, 2 out]
          n524 = property on="Pump Settings" class="Clust (strict)"("Visible"=w1087) -> ()  [unwired: 2 in, 2 out]
        }
      }
      "Progress Out" <- w33
      "CalStatus Out" <- w31
      n525 = local read "time_now"() -> (w29:timestamp)
      n526 = local read "start time"() -> (w30:timestamp)
      n527 = Subtract(x=w29, y=w30) -> (x-y=→"elapsed time":dbl)
      n528 = local write "Progress"(w33) -> ()
    }
    frame #2 {
    }
  }
